vi "Main.vi"() -> ()   [LabVIEW 2012]
doc: "The top-level, or parent, VI for the Advanced Beam Line Electronics (ABLE) application. This VIs also acts as the main graphical user interface (GUI) for the application."
uses:
  ExperimentRun.ctl
  ExperimentRunTiming.ctl
  ExperimentRunDose.ctl
  ExperimentRunFluence.ctl
  ExperimentRunTotalCharge.ctl
  TemperatureAlarmSetup.ctl
  TemperatureAlarmStatus.ctl
  AboutButton.ctl
  UIActionQueueElement.ctl
  UIAction.ctl
  ExperimentActionQueueElement.ctl
  ExperimentAction.ctl
  Experiment.ctl
  Sample.ctl
  BeamLine.ctl
  BeamLineType.ctl
  BeamLineIon.ctl
  AlarmSetups.ctl
  AlarmSetup.ctl
  AlarmQueueElement.ctl
  AlarmAction.ctl
  <vilib>/Utility/error.llb/DialogType.ctl
  HardwareActionQueueElement.ctl
  HardwareAction.ctl
  libs/LV-Utilities/LV-Utilities.lvlib
panel:
  in  "SHOW ABOUT":T1
  in  "ALARMS":bool
  out "Runs":T2[](array[typedef])
  in  "EXPERIMENT":bool
  in  "OVERVIEW":bool
  in  "Tab Control":enum32{"Overview", "Experiment", "Alarms"}(tab)
  out "Overview Temperatures":dbl[][](graph)
  out "Overview Currents":dbl[][](graph)
  out "Beam Profile":cluster{"Waveform":dbl[], "Waveform":dbl[]}[](graph)
  out "DPA Rate":dbl format="%.3e"
  out "Flux":dbl format="%.3e"
  out "Average Flux":dbl format="%.3e"
  out "Average DPA Rate":dbl format="%.3e"
  out "Completed":dbl format="%.1f"
  out "Fluence":dbl format="%.3e"
  out "Dose":dbl format="%.3e"
  out "Total Charge":dbl format="%.3p"
  out "West Aperture":dbl format="%.1p"
  out "Beam Current":dbl format="%.1p"
  out "East Aperture":dbl format="%.1p"
  out "South Aperture":dbl format="%.1p"
  out "North Aperture":dbl format="%.1p"
  out "Overview Voltages":dbl(graph)
  out "Total Ion Energy":dbl format="%.3f"
  out "Terminal Voltage":dbl format="%.3p"
  out "Average":dbl format="%.1f"
  out "Temperature 3":dbl format="%.1f"
  out "Temperature 2":dbl format="%.1f"
  out "Temperature 1":dbl format="%.1f"
  out "Experiment Total Runs":u32
  in  "SHOW RUNS":bool
  out "Experiment Completed":dbl=nan format="%.1f"
  in  "Experiment Target Dose (dpa)":dbl=nan format="%.3e"
  in  "Experiment Project":string
  in  "Experiment Operator":string="Operator"
  in  "SELECT SRIM":bool
  in  "Experiment Sample SRIM Damage Peak (disp * ion / cm)":dbl=nan format="%.2e"
  in  "Experiment Beam Line Total Source Ion Energy (kV)":dbl=nan format="%.1f"
  in  "Experiment Beam Line Charge State":u8=1
  in  "Experiment Beam Line Ion":T7(ring)
  in  "Experiment Beam Line Type":T8(ring)
  in  "Experiment Sample Irradiation Area (cm^2)":dbl=nan format="%.4f"
  in  "Experiment Sample Density (g/cm^3)":dbl=nan format="%.3f"
  in  "Experiment Sample Molar Mass (g/mol)":dbl=nan format="%.3f"
  in  "Experiment Sample Name":string="Sample Name"
  in  "Experiment Sample Description":string="Sample Description"
  out "Experiment File Path":path
  out "Running?":bool
  in  "START EXPERIMENT":bool
  in  "CLOSE EXPERIMENT":bool
  in  "SAVE EXPERIMENT":bool
  in  "OPEN EXPERIMENT":bool
  in  "NEW EXPERIMENT":bool
  out "Temperature 2 Alarm Status":T9={"Actual (C)"=nan, "Activated?"=FALSE} {"Actual (C)" format="%.1f"}
  in  "Temperature 2 Alarm Setup":T10={"ENABLED"=FALSE, "High Limit (C)"=nan, "Low Limit (C)"=nan} {"Low Limit (C)" format="%.1f"; "High Limit (C)" format="%.1f"}
  out "Temperature 1 Alarm Status":T9={"Actual (C)"=nan, "Activated?"=FALSE} {"Actual (C)" format="%.1f"}
  in  "Temperature 1 Alarm Setup":T10={"ENABLED"=FALSE, "High Limit (C)"=nan, "Low Limit (C)"=nan} {"Low Limit (C)" format="%.1f"; "High Limit (C)" format="%.1f"}
  in  "Average Temperature Alarm Setup":T10={"ENABLED"=FALSE, "High Limit (C)"=nan, "Low Limit (C)"=nan} {"Low Limit (C)" format="%.1f"; "High Limit (C)" format="%.1f"}
  out "Average Temperature Alarm Status":T9={"Actual (C)"=nan, "Activated?"=FALSE} {"Actual (C)" format="%.1f"}
  in  "Temperature 3 Alarm Setup":T10={"ENABLED"=FALSE, "High Limit (C)"=nan, "Low Limit (C)"=nan} {"Low Limit (C)" format="%.1f"; "High Limit (C)" format="%.1f"}
  out "Temperature 3 Alarm Status":T9={"Actual (C)"=nan, "Activated?"=FALSE} {"Actual (C)" format="%.1f"}
  in  "DONE":bool
  # "Experiment"
  # "Currents"
  # "Voltages"
  # "Temperatures"
  # "RUNS"
  # "Total Runs"
  # "Completed (%)"
  # "Experiment"
  # "Target Dose"
  # "Project Description"
  # "Operator"
  # "SRIM"
  # "Damage Peak (D1)"
  # "Beam Line"
  # "Total Source Ion Energy"
  # "Ion"
  # "+"
  # "Type"
  # "Sample"
  # "Irradiation Area"
  # "Density"
  # "Molar Mass"
  # "Name"
  # "Description"
  # "Temperature 2"
  # "Actual"
  # "Low Limit"
  # "High Limit"
  # "Temperature 1"
  # "Actual"
  # "Low Limit"
  # "High Limit"
  # "Average Temperature"
  # "Low Limit"
  # "High Limit"
  # "Actual"
  # "Temperature 3"
  # "Low Limit"
  # "High Limit"
  # "Actual"
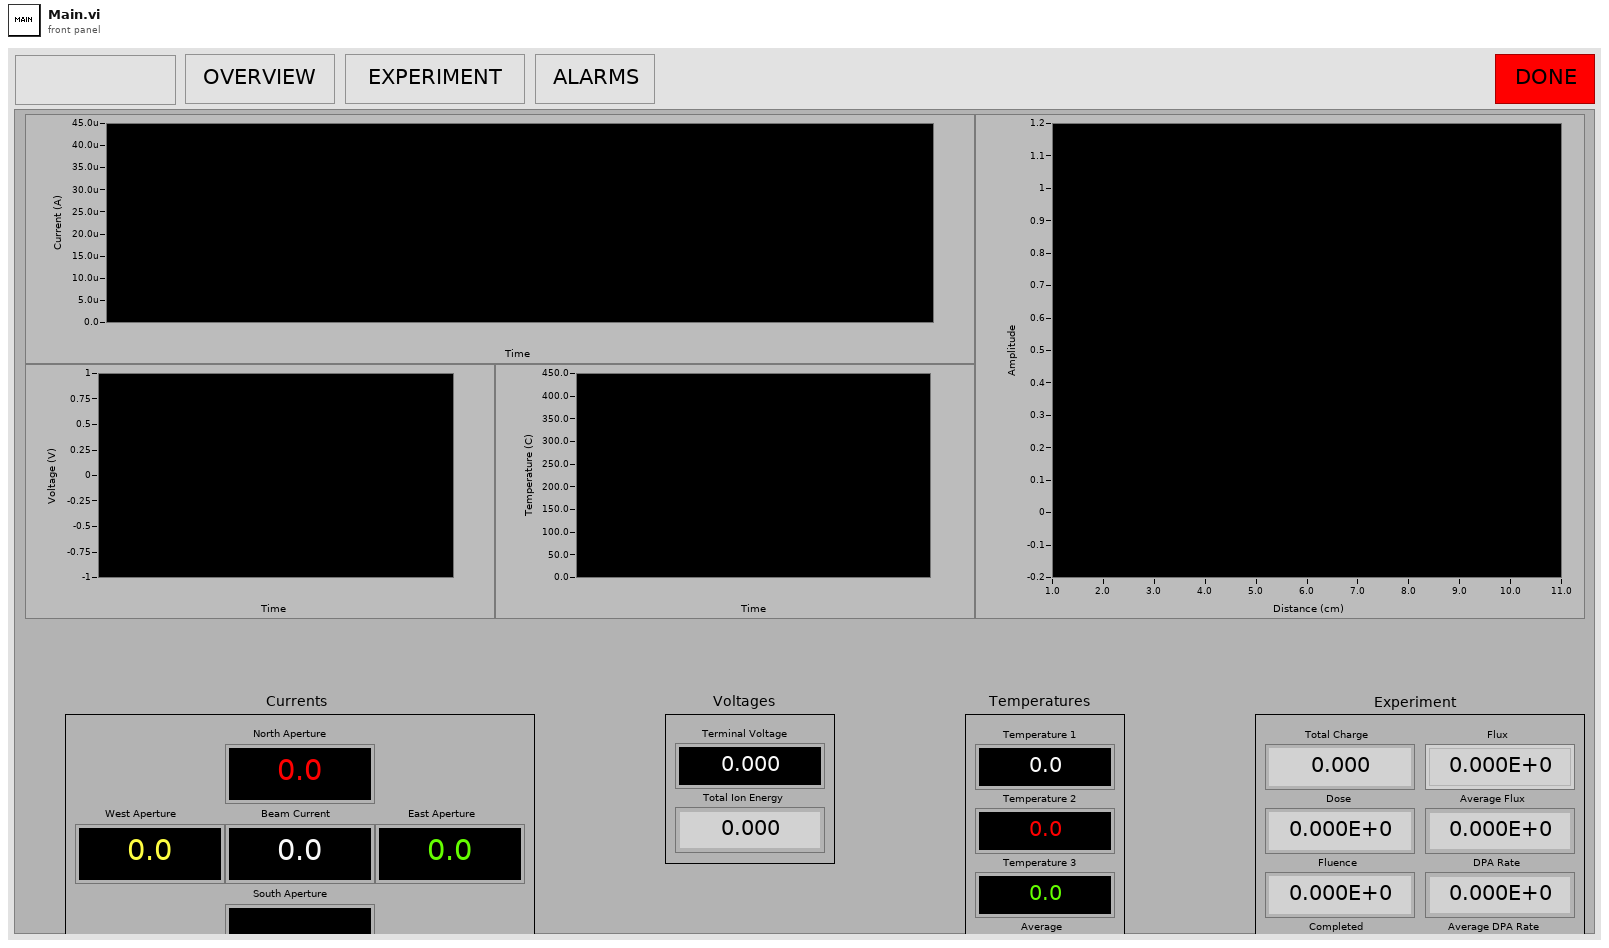
[diagram p1: front panel]
types:
  T1 = typedef "AboutButton.ctl" = bool
  T2 = typedef "ExperimentRun.ctl" = cluster{"Timing":T3, "Dose (dpa)":T4, "Fluence (ions/cm^2)":T5, "Total Charge (C)":T6}
  T3 = typedef "ExperimentRunTiming.ctl" = cluster{"Start":timestamp, "Stop":timestamp}
  T4 = typedef "ExperimentRunDose.ctl" = cluster{"Start":dbl, "Stop":dbl}
  T5 = typedef "ExperimentRunFluence.ctl" = cluster{"Start":dbl, "Stop":dbl}
  T6 = typedef "ExperimentRunTotalCharge.ctl" = cluster{"Start":dbl, "Stop":dbl}
  T7 = enum16{"H", "He", "C", "Fe", "Ni", "Pt", "Si", "Ag", "Au"}
  T8 = enum16{"Ion Beam Analysis", "Auxiliary", "Radiation Damage"}
  T9 = typedef "TemperatureAlarmStatus.ctl" = cluster{"Actual (C)":dbl, "Activated?":bool}
  T10 = typedef "TemperatureAlarmSetup.ctl" = cluster{"ENABLED":bool, "High Limit (C)":dbl, "Low Limit (C)":dbl}
  T11 = typedef "ABLEConfiguration.ctl" = cluster{"Display":T12, "Simulate Data?":bool, "Folder":T13, "Alarms":T14, "Keithley 6485":T15, "Keithley 6482":T16}
  T12 = typedef "DisplayConfiguration.ctl" = cluster{"Defualt Monitor":u16, "Center on Monitor?":bool, "Hardware Display Period (msec)":u32, "Experiment Display Period (msec)":u32}
  T13 = typedef "FolderConfiguration.ctl" = cluster{"Hardware Log":path, "Experiment Log":path, "Experiment":path, "SRIM Simulation":path}
  T14 = typedef "AlarmsConfiguration.ctl" = cluster{"Temperature Alarm Sound File":path, "Temperature Alarm Sound Delay (sec)":dbl}
  T15 = typedef "Keithley6485Configuration.ctl" = cluster{"GPIB IDs":u8[], "GPIB Board IDs":u8[], "Display On?":bool[], "Integration Rates":dbl[], "Auto Range?":bool[], "Ranges (A)":dbl[]}
  T16 = typedef "Keithley6482Configuration.ctl" = cluster{"GPIB IDs":u8[], "GPIB Board IDs":u8[], "Display On?":bool[], "Integration Rates":dbl[], "Auto Range?":bool[], "Ranges (A)":dbl[]}
  T17 = typedef "ABLEDataStructures.ctl" = cluster{"Hardware Display":refnum<notifier>, "BPM":refnum<notifier>, "Experiment Hardware":refnum<notifier>, "Experiment Display":refnum<notifier>, "Alarm Display":refnum<notifier>}
  T18 = typedef "ActionQueues.ctl" = cluster{"UI Action":refnum<queue>, "Hardware Action":refnum<queue>, "Experiment Action":refnum<queue>, "Alarm Action":refnum<queue>}
  T19 = typedef "HardwareDisplayData.ctl" = cluster{"Temperatures (C)":dbl[], "Terminal Voltage (MeV)":dbl, "Currents (A)":dbl[]}
  T20 = typedef "AlarmData.ctl" = cluster{"Temperature":T21[]}
  T21 = typedef "AlarmDatum.ctl" = cluster{"Actual":dbl, "Activated?":bool}
  T22 = typedef "ExperimentData.ctl" = cluster{"Flux (ions/s * cm^2)":dbl, "Average Flux (ions/s * cm^2)":dbl, "DPA Rate":dbl, "Average DPA Rate":dbl, "Total Ion Energy (MeV)":dbl, "Total Charge (C)":dbl, "Dose (DPA)":dbl, "Fluence (ions/cm^2)":dbl, "Percent Complete (%)":dbl, "Duration (sec)":dbl}
  T23 = typedef "UIActionQueueElement.ctl" = cluster{"Action":T24, "Data":variant}
  T24 = typedef "UIAction.ctl" = enum16{"Initalize", "Create Experiment", "Created", "Read Experiment Controls", "Read Alarm Controls", "Loaded", "Save Experiment", "Saved", "Write Experiment Controls", "Read Experiment", "Read", "Start Experiment", "Started", "Stop Experiment", "Stopped", "Close Experiment", "Closed", "SRIM", "Error", "Shutdown"}
  T25 = enum8{"Enabled", "Disabled", "Disabled and Grayed Out"}
  T26 = typedef "ExperimentActionQueueElement.ctl" = cluster{"Action":T27, "Data":variant}
  T27 = typedef "ExperimentAction.ctl" = enum16{"Initialize", "Create", "Read", "Load", "Start", "Run", "Stop", "Save", "Shutdown"}
  T28 = typedef "BeamLine.ctl" = cluster{"Type":T29, "Ion":T30, "Charge State":u8, "Total Source Ion Energy (kV)":dbl}
  T29 = typedef "BeamLineType.ctl" = enum16{"Ion Beam Analysis", "Auxiliary", "Radiation Damage"}
  T30 = typedef "BeamLineIon.ctl" = enum16{"H", "He", "C", "Fe", "Ni", "Pt", "Si", "Ag", "Au"}
  T31 = typedef "Sample.ctl" = cluster{"Name":string, "Description":string, "Molar Mass (g/mol)":dbl, "Density (g/cm^3)":dbl, "Irradiation Area (cm^2)":dbl, "SRIM Damage Peak (disp * ions/cm)":dbl}
  T32 = typedef "Experiment.ctl" = cluster{"File Path":path, "Operator":string, "Project":string, "Target Dose (dpa)":dbl, "Sample":T31, "Beam Line":T28, "Runs":T2[]}
  T33 = typedef "AlarmQueueElement.ctl" = cluster{"Action":T34, "Data":variant}
  T34 = typedef "AlarmAction.ctl" = enum16{"Initialize", "Load", "Check", "Shutdown"}
  T35 = typedef "AlarmSetups.ctl" = cluster{"Temperature":T36[]}
  T36 = typedef "AlarmSetup.ctl" = cluster{"ENABLED":bool, "High Limit":dbl, "Low Limit":dbl}
  T37 = typedef "HardwareActionQueueElement.ctl" = cluster{"Action":T38, "Data":variant}
  T38 = typedef "HardwareAction.ctl" = enum16{"Initialize", "Collect", "Shutdown"}
  T39 = typedef "DialogType.ctl" = u16
  T40 = typedef "BPM.ctl" = cluster{dbl[], "Beam Profile":dbl[]}[]
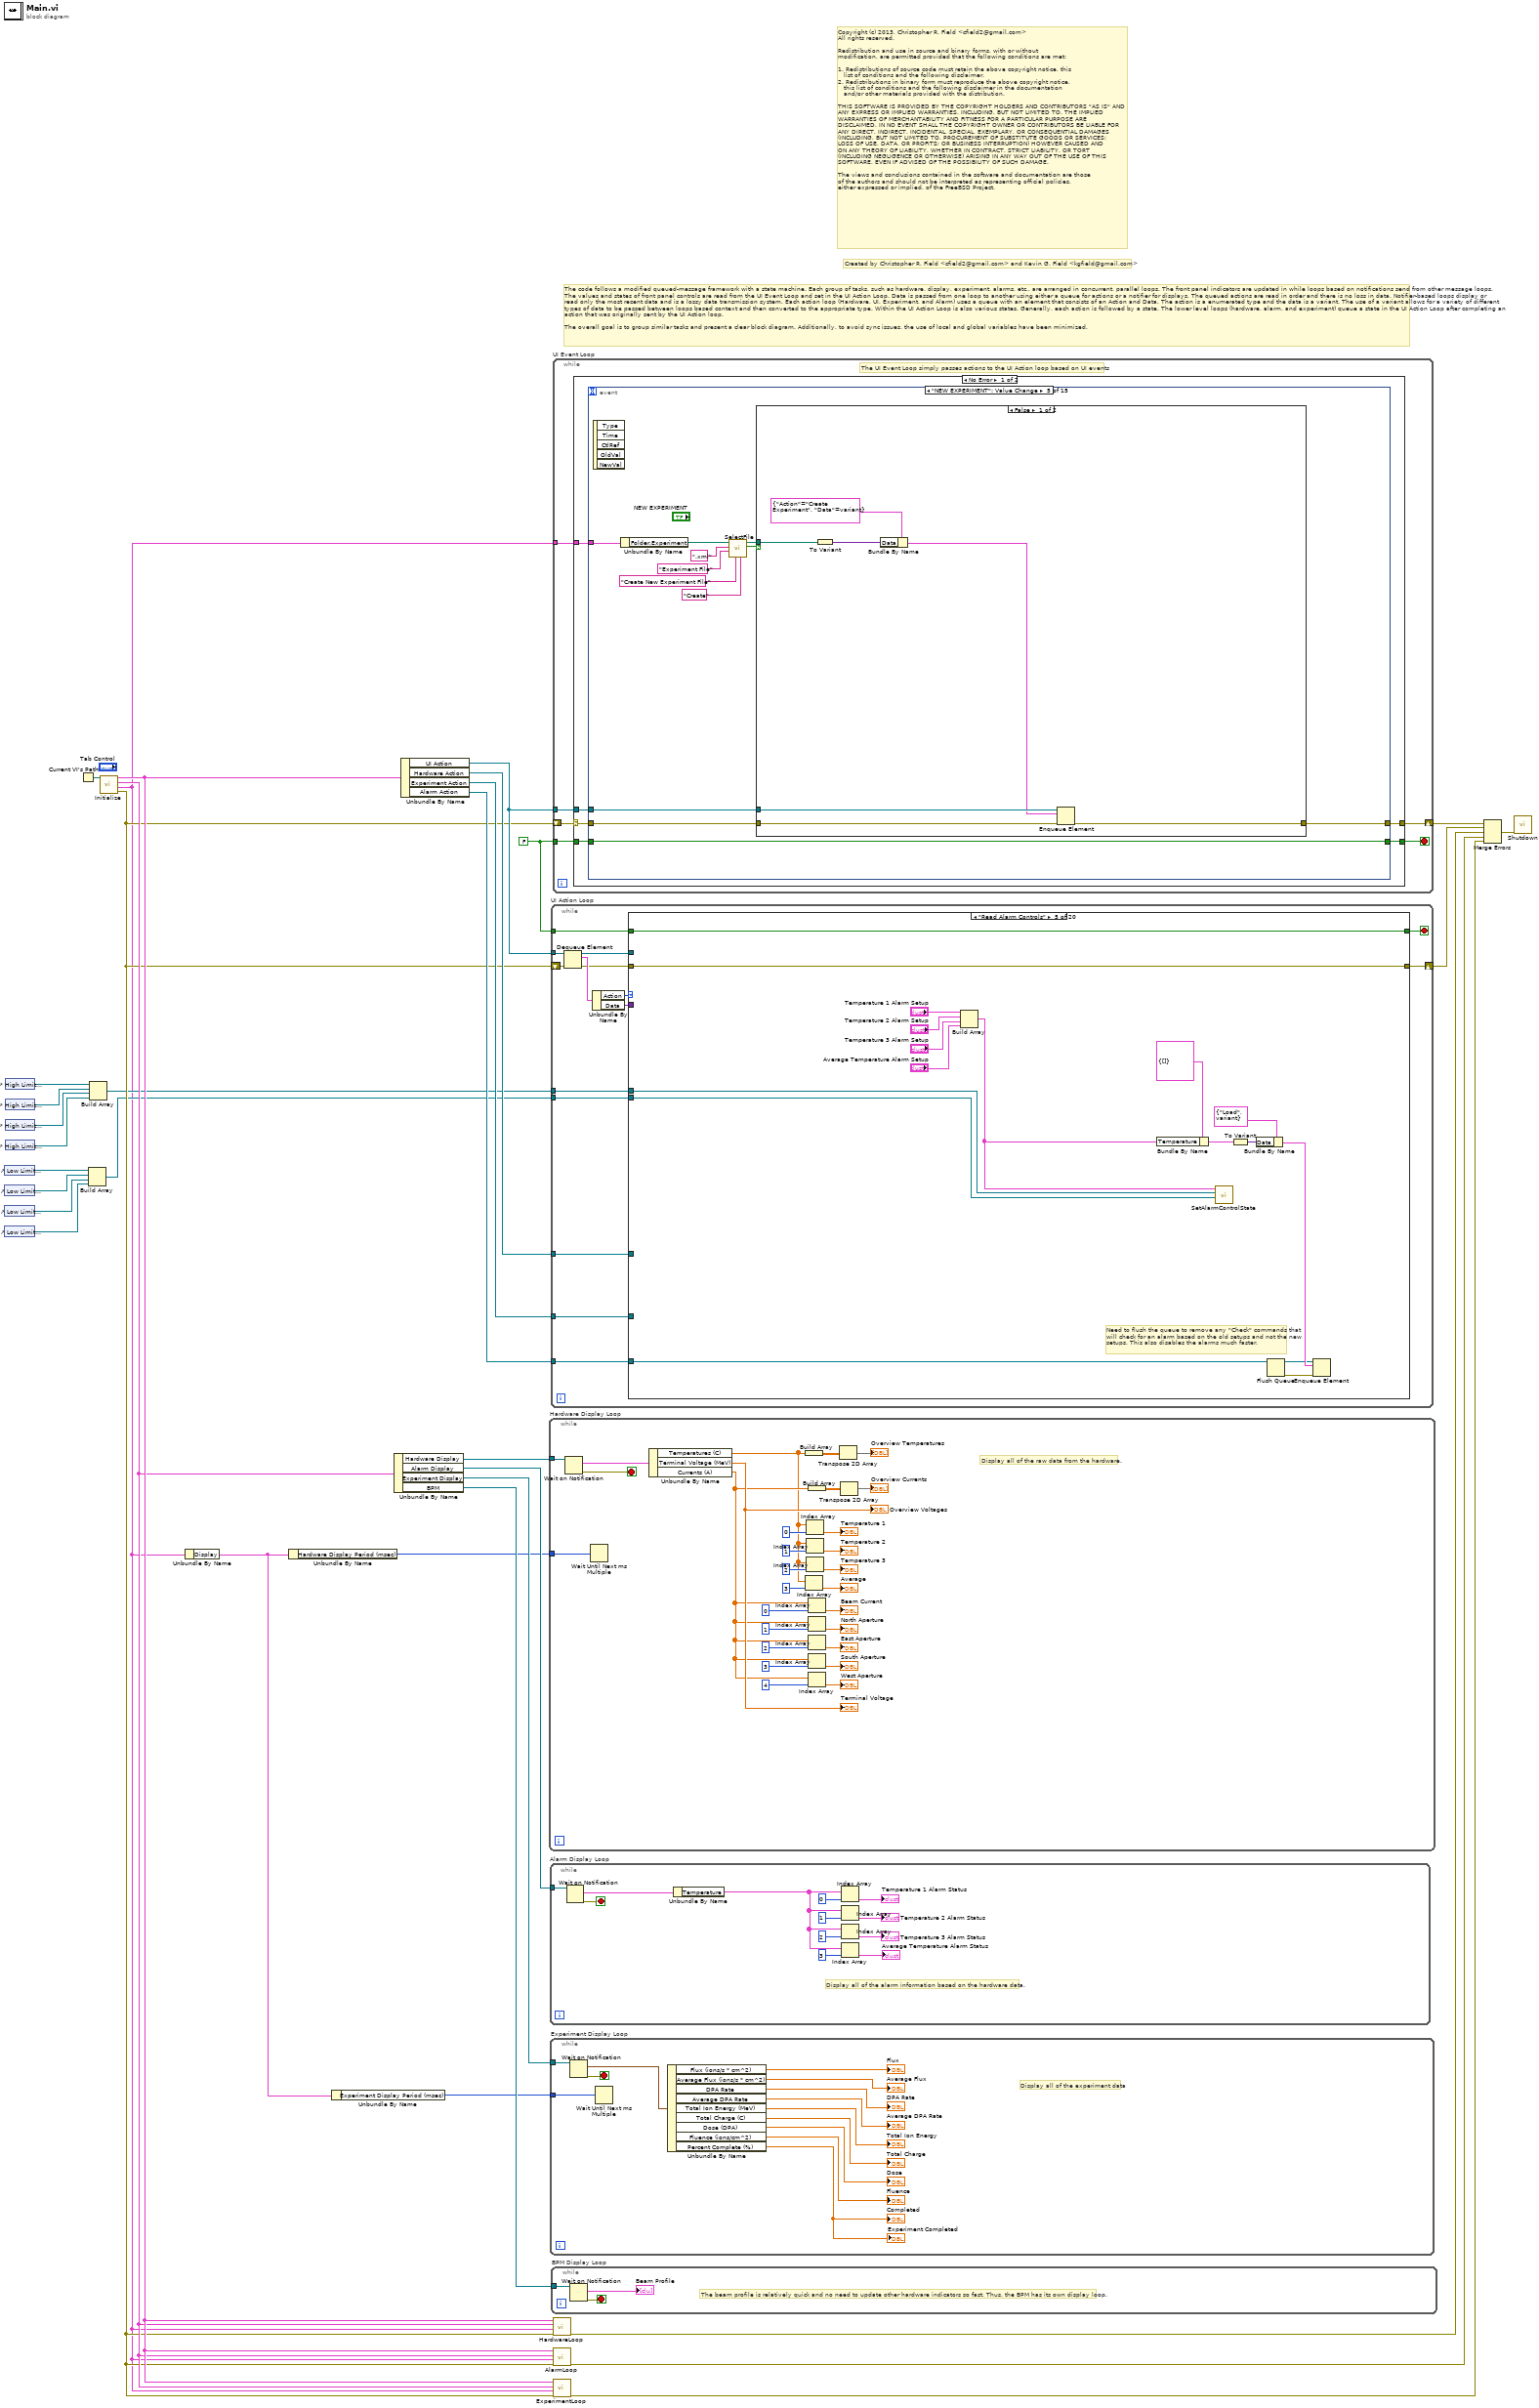
[diagram p0: block diagram]
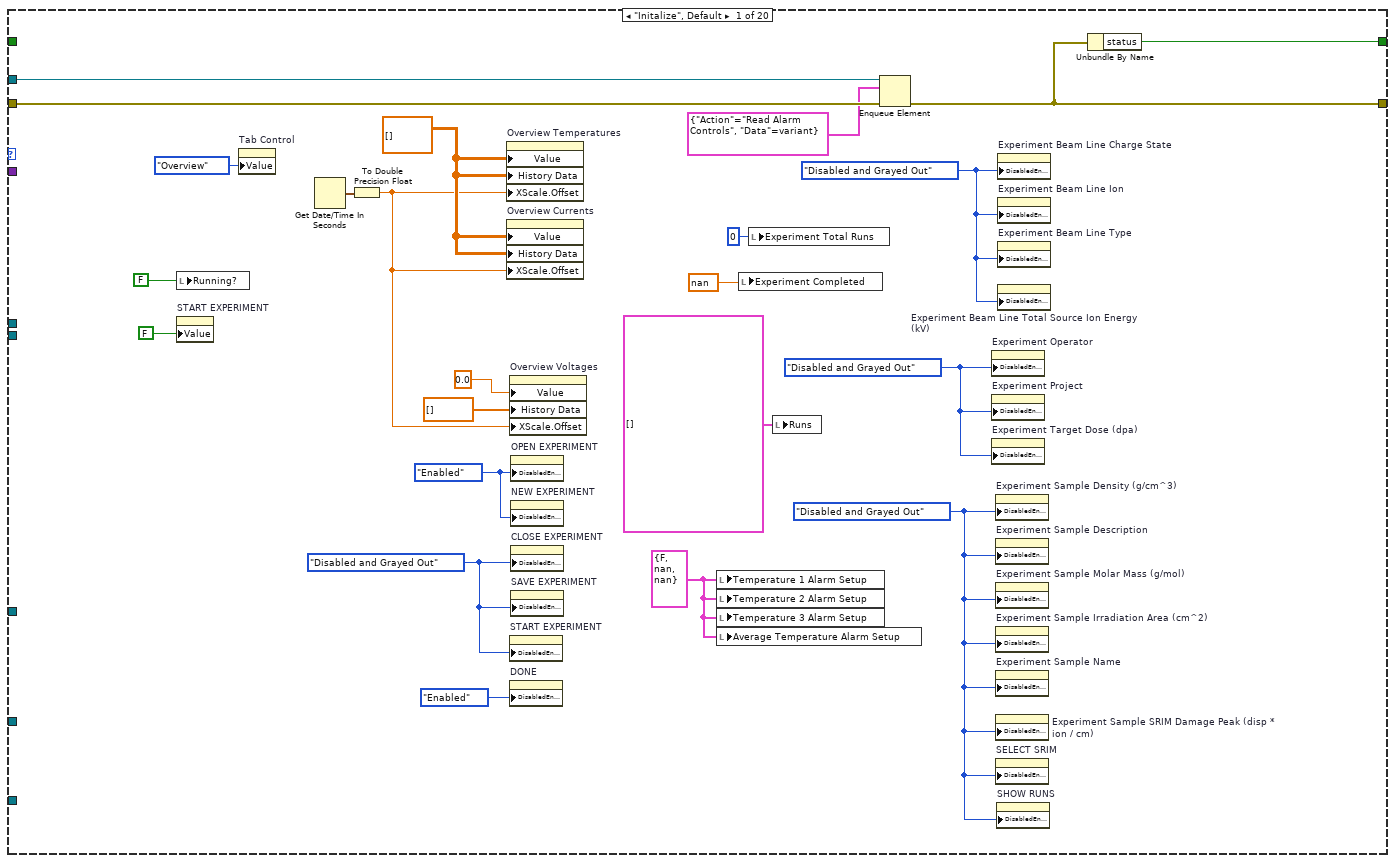
[diagram p2: hidden frame]
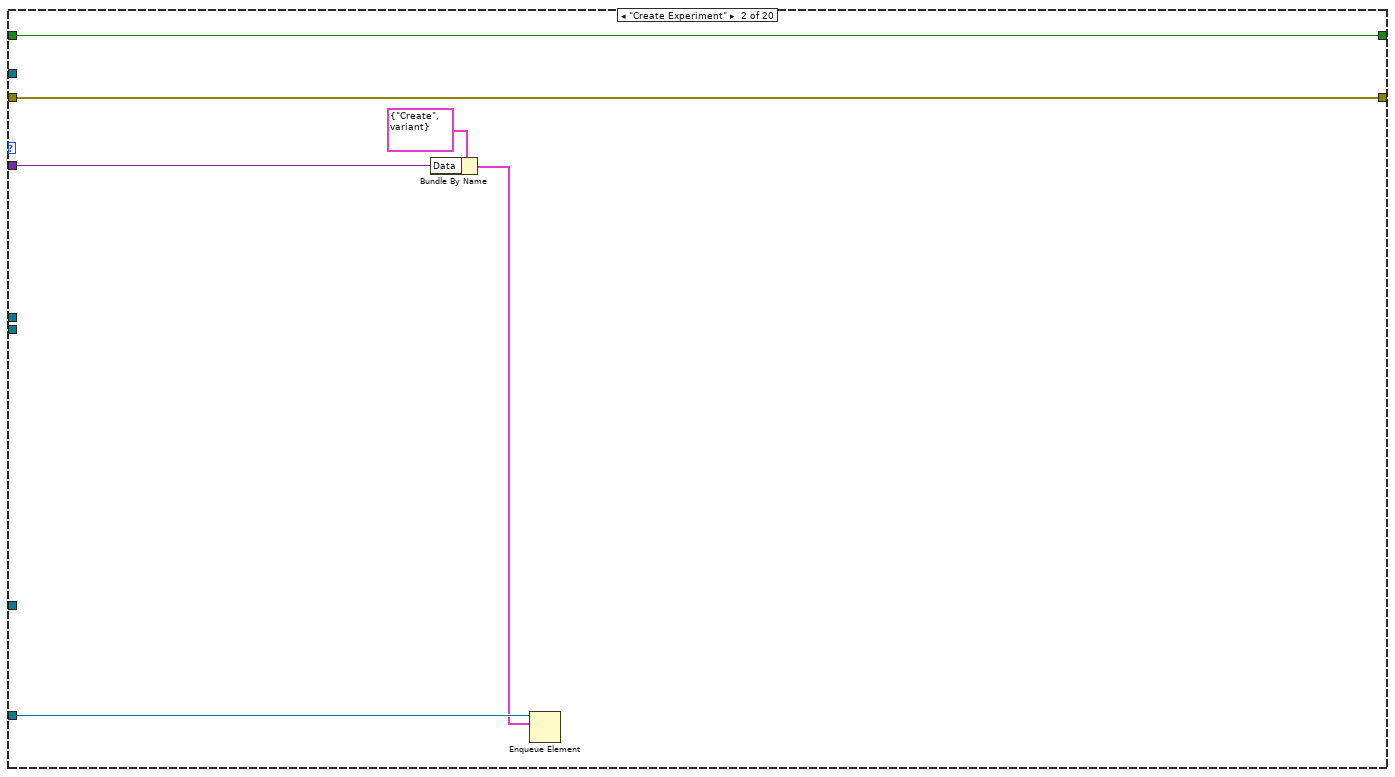
[diagram p3: hidden frame]
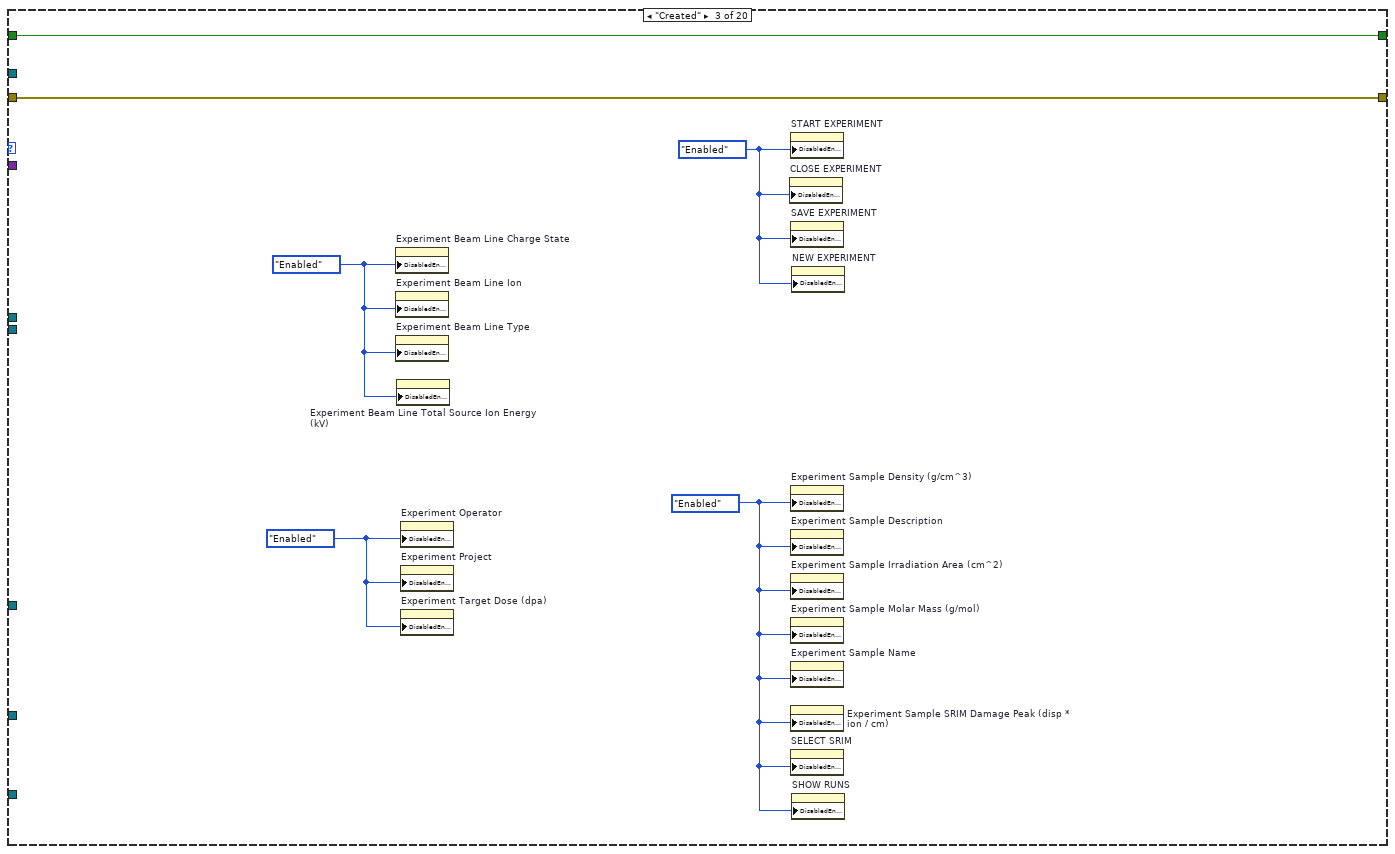
[diagram p4: hidden frame]
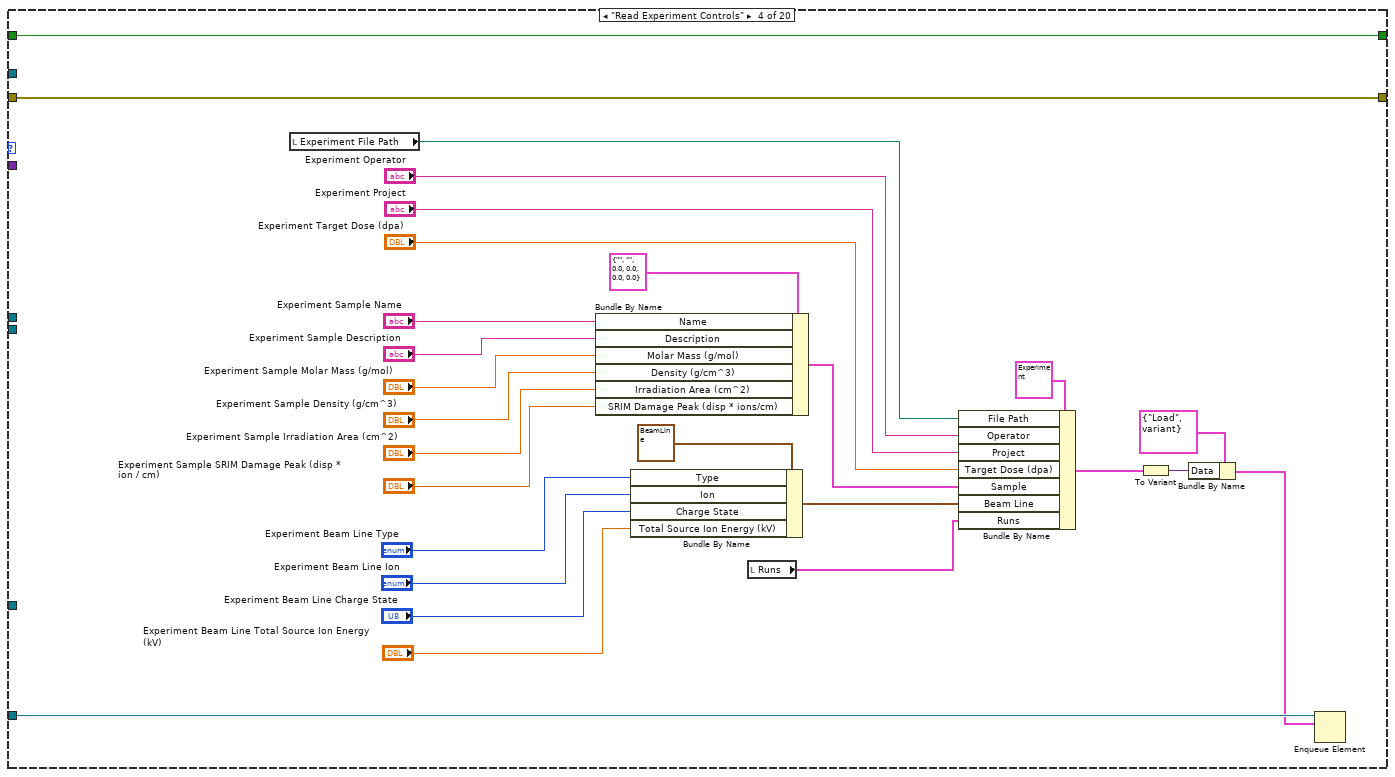
[diagram p5: hidden frame]
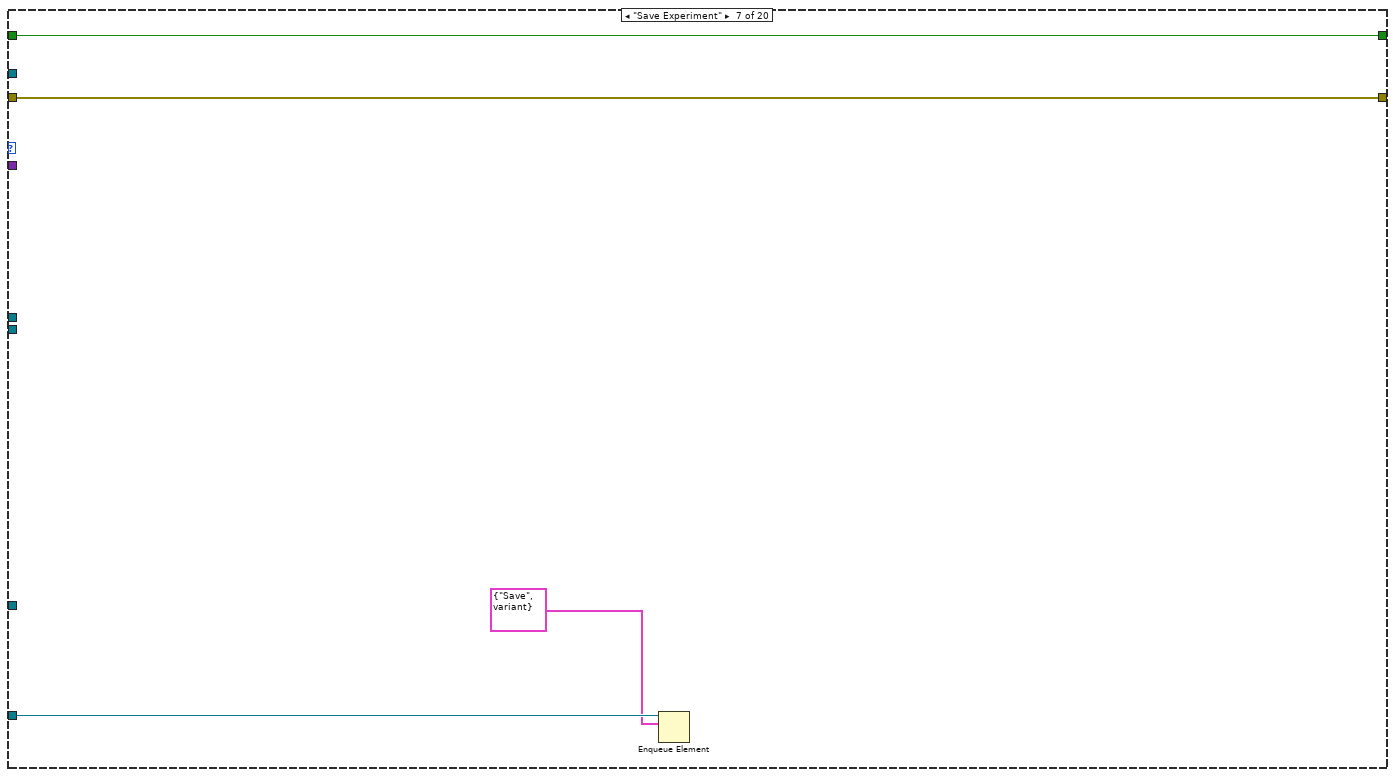
[diagram p7: hidden frame]
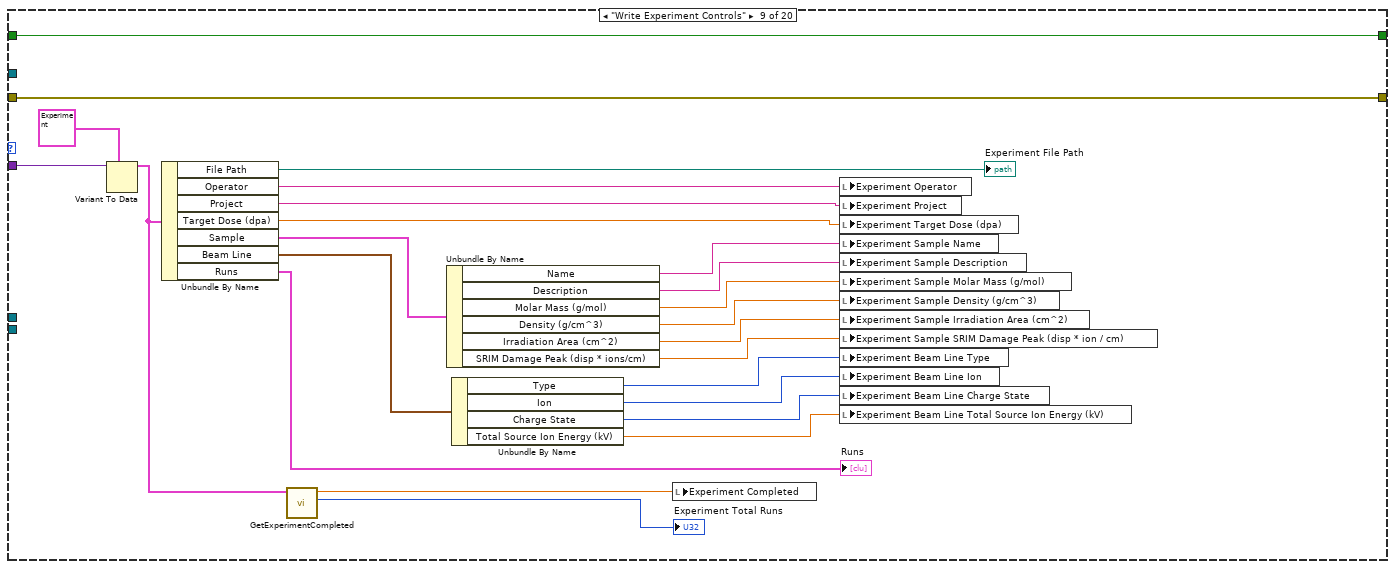
[diagram p9: hidden frame]
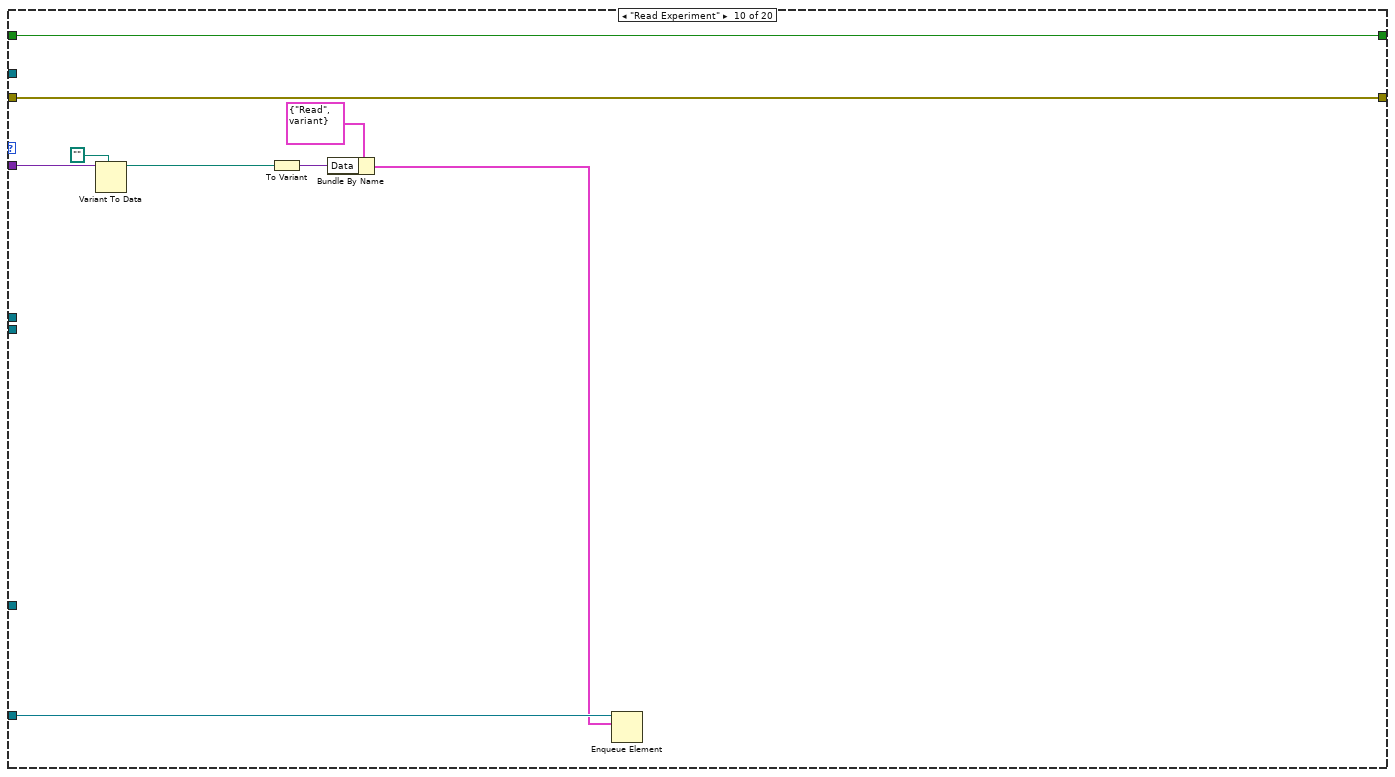
[diagram p10: hidden frame]
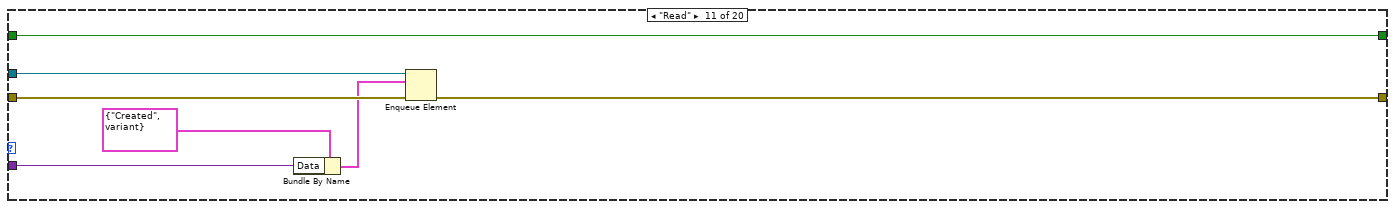
[diagram p11: hidden frame]
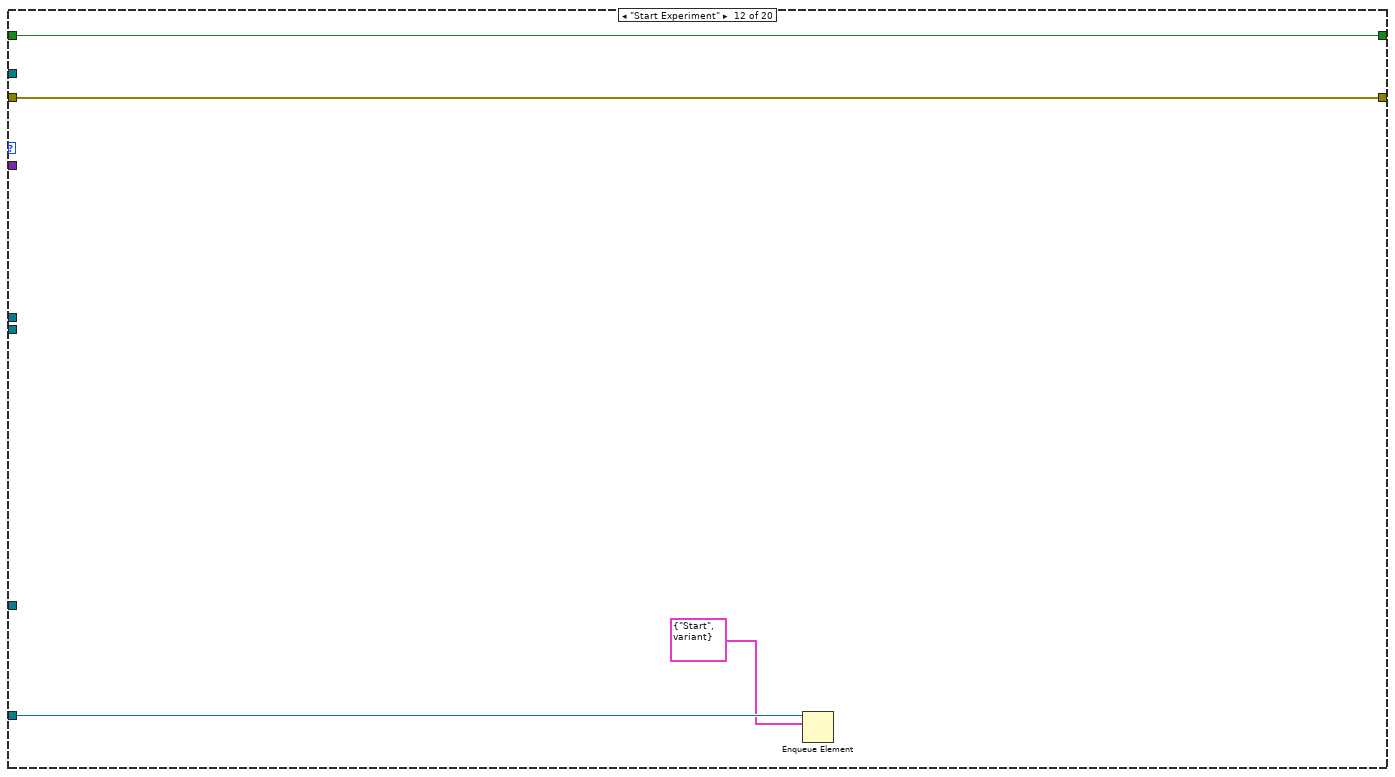
[diagram p12: hidden frame]
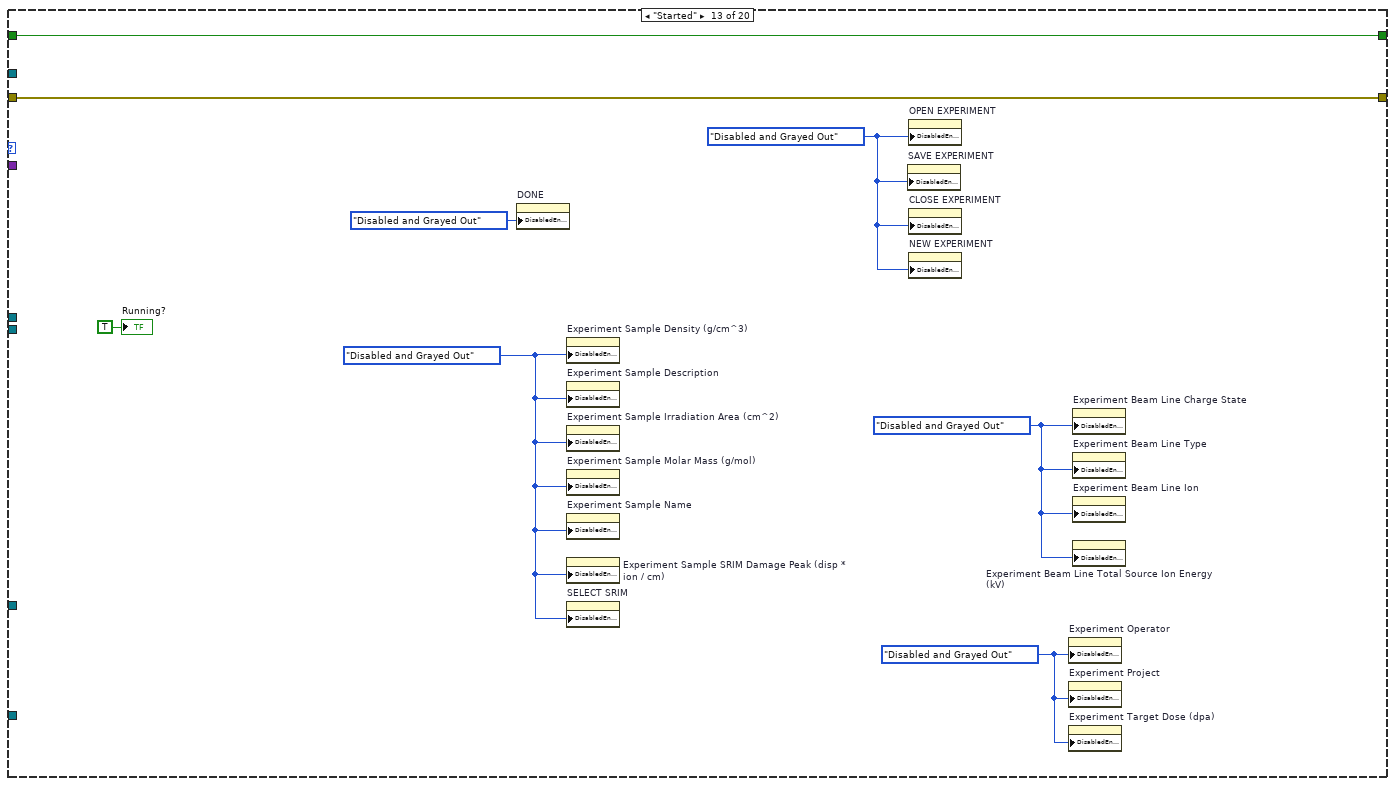
[diagram p13: hidden frame]
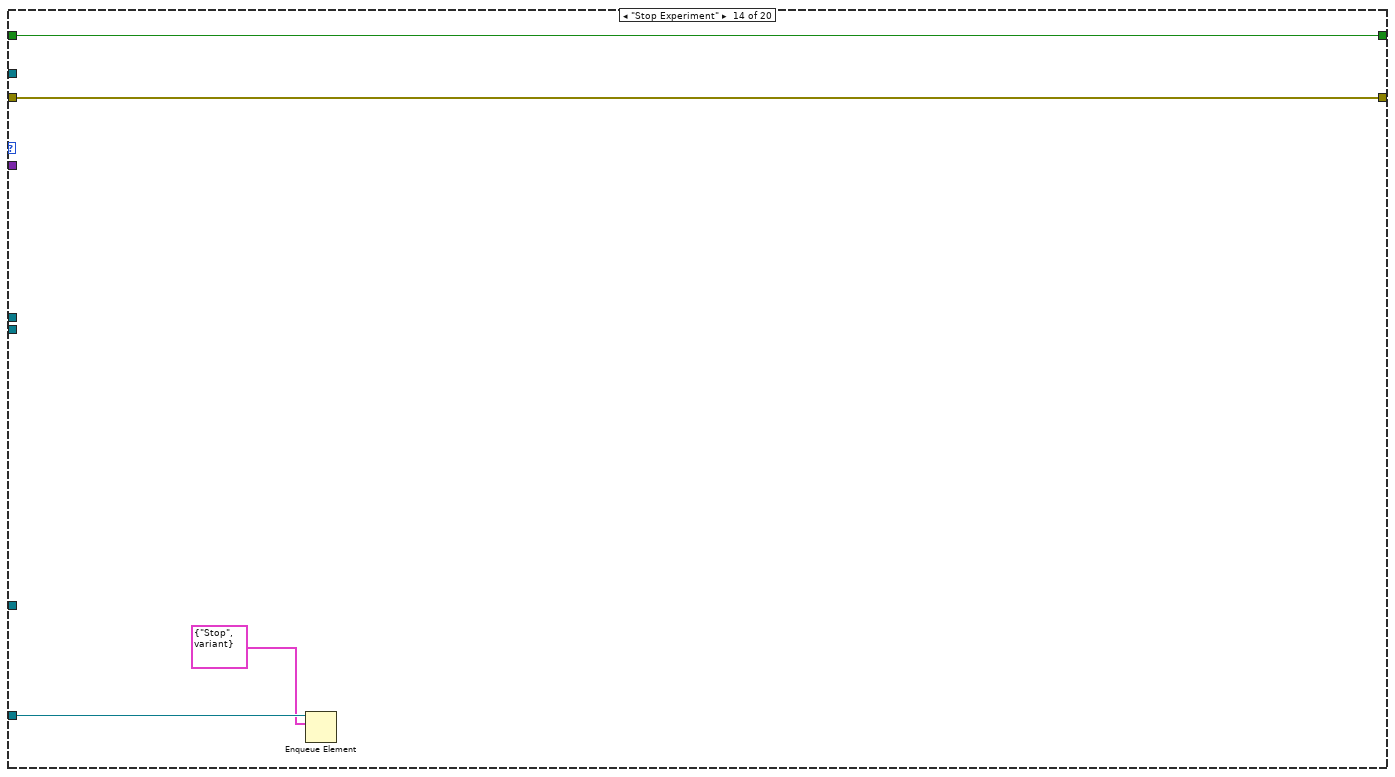
[diagram p14: hidden frame]
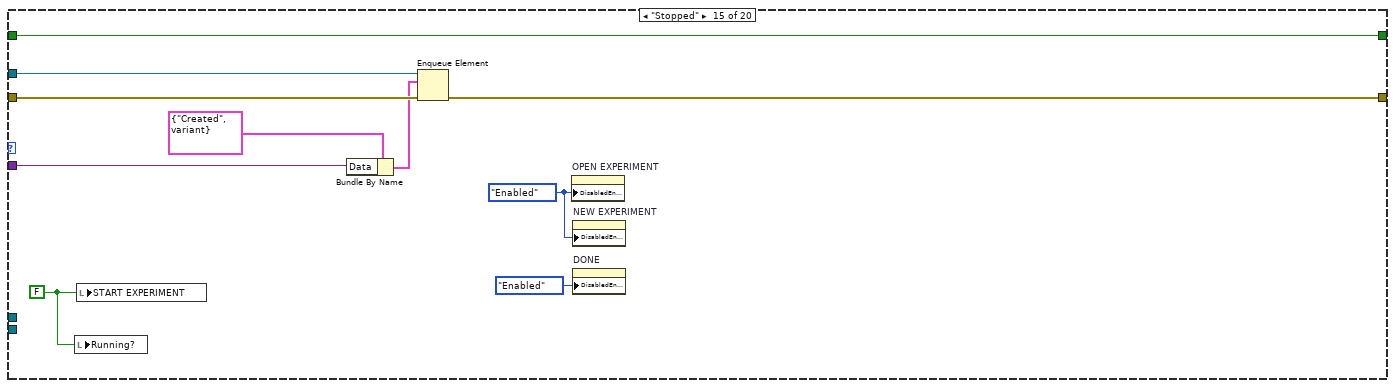
[diagram p15: hidden frame]
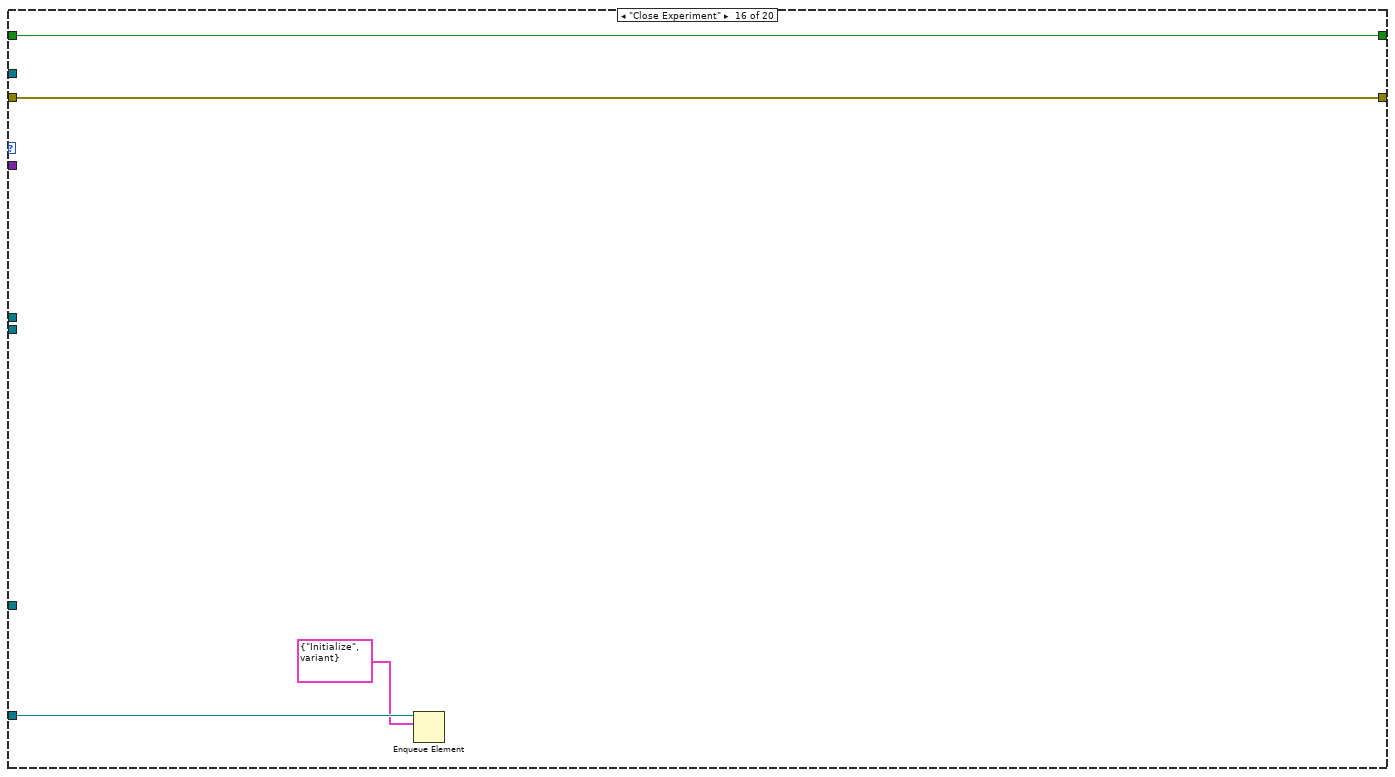
[diagram p16: hidden frame]
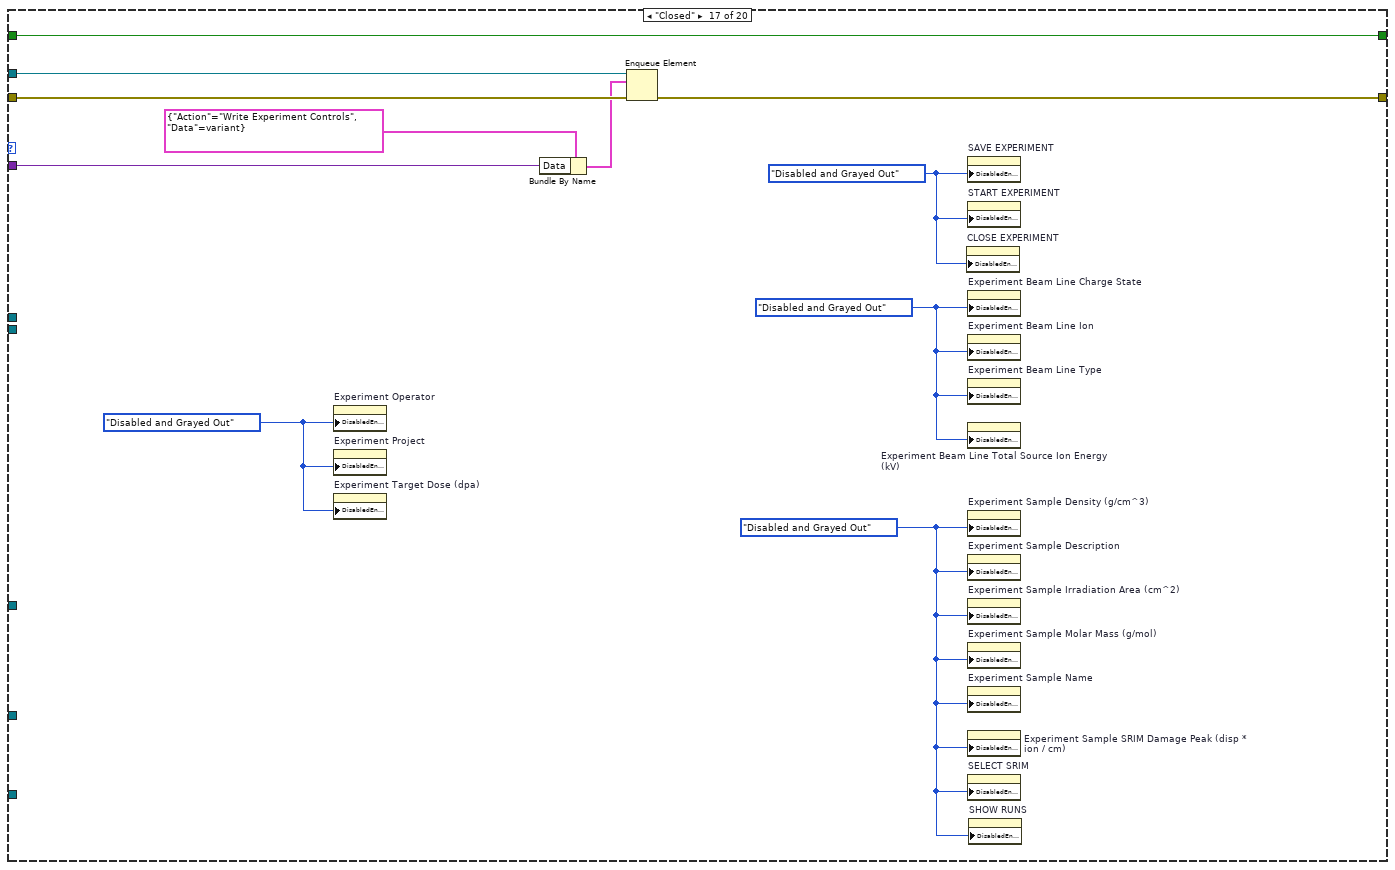
[diagram p17: hidden frame]
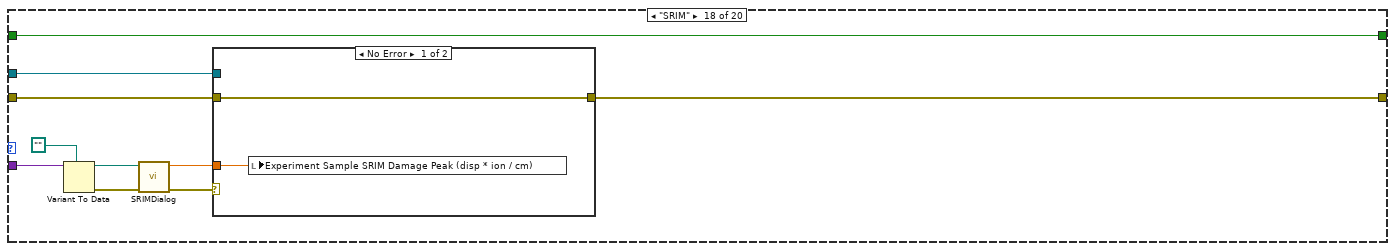
[diagram p18: hidden frame]
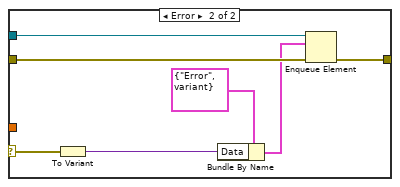
[diagram p19: hidden frame]
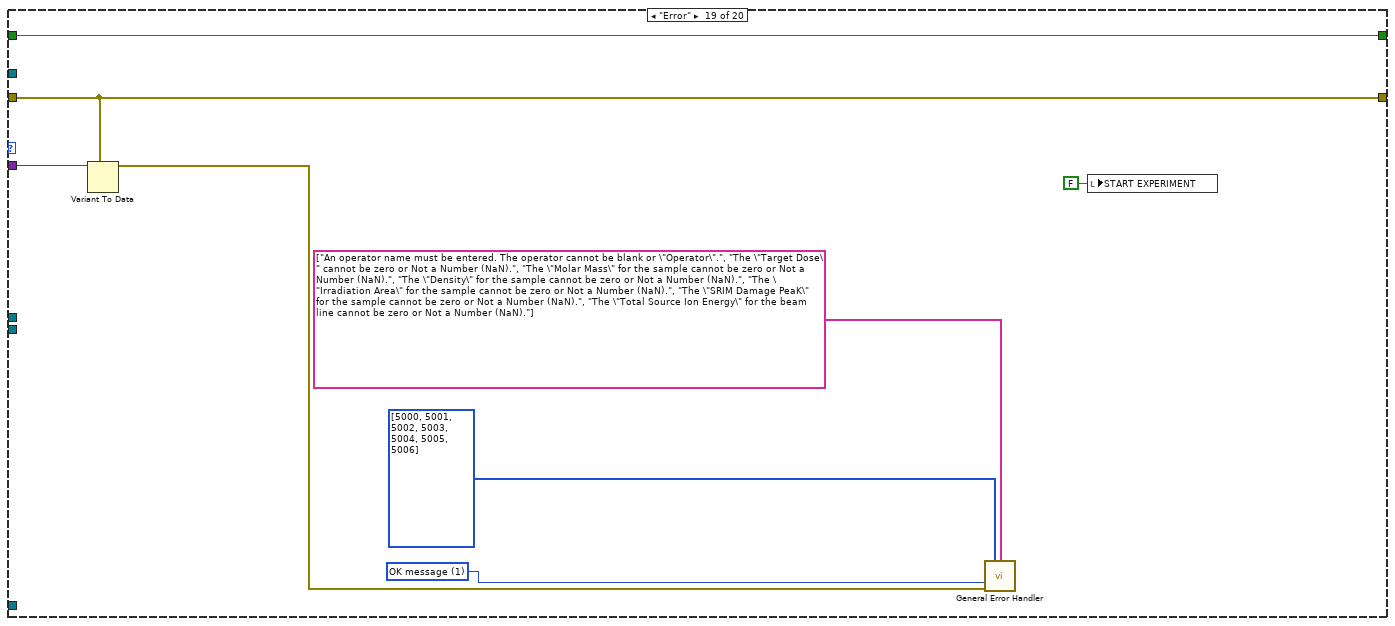
[diagram p20: hidden frame]
diagram:
  w33 = FALSE
  # "Copyright (c) 2013, Christopher R. Field <cfield2@gmail.com>\nAll rights reserved.\n\nRedistribution and use in source and binary forms, with or without\nmodification, are permitted provided that the following conditions are met: \n\n1. Redistributions of source code must retain the above copyright notice, this\n   list of conditions and the following disclaimer. \n2. Redistributions in binary form must reproduce the above copyright notice,\n   this list of conditions and the following disclaimer in the documentation\n   and/or other materials provided with the distribution. \n\nTHIS SOFTWARE IS PROVIDED BY THE COPYRIGHT HOLDERS AND CONTRIBUTORS \"AS IS\" AND\nANY EXPRESS OR IMPLIED WARRANTIES, INCLUDING, BUT NOT LIMITED TO, THE IMPLIED\nWARRANTIES OF MERCHANTABILITY AND FITNESS FOR A PARTICULAR PURPOSE ARE\nDISCLAIMED. IN NO EVENT SHALL THE COPYRIGHT OWNER OR CONTRIBUTORS BE LIABLE FOR\nANY DIRECT, INDIRECT, INCIDENTAL, SPECIAL, EXEMPLARY, OR CONSEQUENTIAL DAMAGES\n(INCLUDING, BUT NOT LIMITED TO, PROCUREMENT OF SUBSTITUTE GOODS OR SERVICES;\nLOSS OF USE, DATA, OR PROFITS; OR BUSINESS INTERRUPTION) HOWEVER CAUSED AND\nON ANY THEORY OF LIABILITY, WHETHER IN CONTRACT, STRICT LIABILITY, OR TORT\n(INCLUDING NEGLIGENCE OR OTHERWISE) ARISING IN ANY WAY OUT OF THE USE OF THIS\nSOFTWARE, EVEN IF ADVISED OF THE POSSIBILITY OF SUCH DAMAGE.\n\nThe views and conclusions contained in the software and documentation are those\nof the authors and should not be interpreted as representing official policies, \neither expressed or implied, of the FreeBSD Project."
  # "Created by Christopher R. Field <cfield2@gmail.com> and Kevin G. Field <kgfield@gmail.com>"
  # "The code follows a modified queued-message framework with a state machine. Each group of tasks, such as hardware, display, experiment, alarms, etc., are arranged in concurrent, parallel loops. The front panel indicators are updated in while loops based on notifications send from other message loops. The values and states of front panel controls are read from the UI Event Loop and set in the UI Action Loop. Data is passed from one loop to another using either a queue for actions or a notifier for displays. The queued actions are read in order and there is no loss in data. Notifier-based loops display or read only the most recent data and is a lossy data transmission system. Each action loop (Hardware, UI, Experiment, and Alarm) uses a queue with an element that consists of an Action and Data. The action is a enumerated type and the data is a variant. The use of a variant allows for a variety of different types of data to be passed between loops based context and then converted to the appropriate type. Within the UI Action Loop is also various states. Generally, each action is followed by a state. The lower level loops (hardware, alarm, and experiment) queue a state in the UI Action Loop after completing an action that was originally sent by the UI Action loop.\n\nThe overall goal is to group similar tasks and present a clear block diagram. Additionally, to avoid sync issues, the use of local and global variables have been minimized."
  n1 = control-ref of="Low Limit (C)"() -> (w7:refnum<vi>)
  n2 = control-ref of="Low Limit (C)"() -> (w8:refnum<vi>)
  n3 = control-ref of="Low Limit (C)"() -> (w9:refnum<vi>)
  n4 = control-ref of="Low Limit (C)"() -> (w10:refnum<vi>)
  n5 = control-ref of="High Limit (C)"() -> (w11:refnum<vi>)
  n6 = control-ref of="High Limit (C)"() -> (w12:refnum<vi>)
  n7 = control-ref of="High Limit (C)"() -> (w13:refnum<vi>)
  n8 = control-ref of="High Limit (C)"() -> (w14:refnum<vi>)
  n9 = Current VI's Path() -> (path=w32:path)
  n10 = Build Array(w7, w8, w9, w10) -> (w5:refnum<vi>[])
  n11 = Build Array(w11, w12, w13, w14) -> (w6:refnum<vi>[])
  n12 = call "Initialize.vi"("VI Path"=w32) -> ("Error Out"=w17:errorcluster, "ABLE Configuration"=w4:T11, "ABLE Data Structures"=w18:T17, "Action Queues"=w19:T18)  [unwired: 7 in]
  n13 = Unbundle By Name(w4) -> ("Display"=w2:T12)
  n14 = Unbundle By Name(w2) -> ("Hardware Display Period (msec)"=w3:u32)
  n15 = Unbundle By Name(w2) -> ("Experiment Display Period (msec)"=w1:u32)
  n16 = Unbundle By Name(w18) -> ("Hardware Display"=w22:refnum<notifier>, "Alarm Display"=w21:refnum<notifier>, "Experiment Display"=w24:refnum<notifier>, "BPM"=w23:refnum<notifier>)
  n17 = Unbundle By Name(w19) -> ("UI Action"=w27:refnum<queue>, "Hardware Action"=w26:refnum<queue>, "Experiment Action"=w25:refnum<queue>, "Alarm Action"=w20:refnum<queue>)
  n18 = while "Hardware Display Loop" {
    tunnel: w22 -> [w41]
    tunnel: w3 -> [w34]
    stop <- w36 stop-if-true
    # "Display all of the raw data from the hardware."
    n19 = Wait on Notification(notifier=w41) -> (notification=w62:T19, error out=w36:errorcluster)  [unwired: 3 in, 2 out]
    n20 = Wait Until Next ms Multiple(millisecond multiple=w34) -> ()  [unwired: 1 out]
    n21 = Unbundle By Name(w62) -> ("Temperatures (C)"=w35:dbl[], "Terminal Voltage (MeV)"=→"Overview Voltages" →"Terminal Voltage":dbl, "Currents (A)"=w48:dbl[])
    n22 = Build Array(w35) -> (w50:dbl[][])
    n23 = Index Array(array=w35, index=3) -> (element=→"Average":dbl)
    n24 = Index Array(array=w35, index=0) -> (element=→"Temperature 1":dbl)
    n25 = Index Array(array=w35, index=1) -> (element=→"Temperature 2":dbl)
    n26 = Index Array(array=w35, index=2) -> (element=→"Temperature 3":dbl)
    n27 = Build Array(w48) -> (w47:dbl[][])
    n28 = Index Array(array=w48, index=3) -> (element=→"South Aperture":dbl)
    n29 = Index Array(array=w48, index=4) -> (element=→"West Aperture":dbl)
    n30 = Index Array(array=w48, index=0) -> (element=→"Beam Current":dbl)
    n31 = Index Array(array=w48, index=1) -> (element=→"North Aperture":dbl)
    n32 = Index Array(array=w48, index=2) -> (element=→"East Aperture":dbl)
    n33 = Transpose 2D Array(2D array=w50) -> (transposed array=→"Overview Temperatures":dbl[][])
    n34 = Transpose 2D Array(2D array=w47) -> (transposed array=→"Overview Currents":dbl[][])
  }
  n35 = while "Alarm Display Loop" {
    tunnel: w21 -> [w65]
    stop <- w74 stop-if-true
    # "Display all of the alarm information based on the hardware data."
    n36 = Wait on Notification(notifier=w65) -> (notification=w64:T20, error out=w74:errorcluster)  [unwired: 3 in, 2 out]
    n37 = Unbundle By Name(w64) -> ("Temperature"=w63:T21[])
    n38 = Index Array(array=w63, index=3) -> (element=→"Average Temperature Alarm Status":T21)
    n39 = Index Array(array=w63, index=0) -> (element=→"Temperature 1 Alarm Status":T21)
    n40 = Index Array(array=w63, index=1) -> (element=→"Temperature 2 Alarm Status":T21)
    n41 = Index Array(array=w63, index=2) -> (element=→"Temperature 3 Alarm Status":T21)
  }
  n42 = while "Experiment Display Loop" {
    tunnel: w24 -> [w86]
    tunnel: w1 -> [w75]
    stop <- w87 stop-if-true
    # "Display all of the experiment data"
    n43 = Wait on Notification(notifier=w86) -> (notification=w85:T22, error out=w87:errorcluster)  [unwired: 3 in, 2 out]
    n44 = Wait Until Next ms Multiple(millisecond multiple=w75) -> ()  [unwired: 1 out]
    n45 = Unbundle By Name(w85) -> ("Flux (ions/s * cm^2)"=→"Flux":dbl, "Average Flux (ions/s * cm^2)"=→"Average Flux":dbl, "DPA Rate"=→"DPA Rate":dbl, "Average DPA Rate"=→"Average DPA Rate":dbl, "Total Ion Energy (MeV)"=→"Total Ion Energy":dbl, "Total Charge (C)"=→"Total Charge":dbl, "Dose (DPA)"=→"Dose":dbl, "Fluence (ions/cm^2)"=→"Fluence":dbl, "Percent Complete (%)"=→"Completed" →"Experiment Completed":dbl)
  }
  n46 = while "UI Action Loop" {
    tunnel: w33 -> [w102]
    shift-right: [w94] -> w30
    shift-left: w17 -> [w98]
    tunnel: w27 -> [w93]
    tunnel: w26 -> [w92]
    tunnel: w25 -> [w91]
    tunnel: w20 -> [w90]
    tunnel: w6 -> [w89]
    tunnel: w5 -> [w88]
    stop <- w95 stop-if-true
    n47 = Dequeue Element(queue=w93, error in (no error)=w98) -> (queue out=w97:refnum<queue>, element=w101:T23, error out=w96:errorcluster)  [unwired: 1 in, 1 out]
    n48 = Unbundle By Name(w101) -> ("Action"=w100:T24, "Data"=w99:variant)
    n49 = case shown="\"Read Alarm Controls\"" w100 {
      tunnel: w102 -> [_ w131 w137 w164 w181 w183 w187 w189 w213 w222 w229 w233 w241 w245 w255 w259 w270 w280 w297 w320]
      tunnel: w99 -> [_ w126 _ _ _ _ _ _ w198 w221 w224 _ _ _ w248 _ w265 w279 w296 _]
      tunnel: w97 -> [w106 _ _ _ _ _ _ _ _ _ w228 _ _ _ w252 _ w269 w271 _ w311]
      tunnel: w96 -> [w105 w130 w133 w162 w180 w182 w186 w188 w212 w219 w227 w232 w235 w243 w250 w258 w268 w273 w295 w310]
      tunnel: [w107 w131 w137 w164 w181 w183 w187 w189 w213 w222 w229 w233 w241 w245 w255 w259 w270 w280 w297 w319] -> w95
      tunnel: [w104 w130 w133 w162 w180 w182 w186 w188 w212 w219 w226 w232 w235 w243 w251 w258 w267 w272 w295 w309] -> w94
      tunnel: w92 -> [_ _ _ _ _ _ _ _ _ _ _ _ _ _ _ _ _ _ _ w308]
      tunnel: w91 -> [_ w129 _ w163 _ _ w185 _ _ w218 _ w231 _ w244 _ w257 _ _ _ w306]
      tunnel: w90 -> [_ _ _ _ w167 _ _ _ _ _ _ _ _ _ _ _ _ _ _ w301]
      tunnel: w89 -> [_ _ _ _ w170 _ _ _ _ _ _ _ _ _ _ _ _ _ _ _]
      tunnel: w88 -> [_ _ _ _ w169 _ _ _ _ _ _ _ _ _ _ _ _ _ _ _]
      frame "Initalize", Default {
        w108 = T10 {"ENABLED"=FALSE, "High Limit (C)"=nan, "Low Limit (C)"=nan} ("Temperature 1 Alarm Setup")
        w110 = T25."Disabled and Grayed Out" ("Disabled")
        w114 = T25."Disabled and Grayed Out" ("Disabled")
        w115 = T25."Disabled and Grayed Out" ("Disabled")
        w116 = T25."Disabled and Grayed Out" ("Disabled")
        w117 = T25."Enabled" ("Disabled")
        w124 = dbl[][] [] ("Currents 2")
        n50 = local write "Running?"(FALSE ("Running?")) -> ()
        n51 = property on="START EXPERIMENT" class="Bool (strict)"("Value"=FALSE ("START EXPERIMENT")) -> ()  [unwired: 2 in, 2 out]
        n52 = property on="Tab Control" class="TabCtl (strict)"("Value"=enum32{"Overview", "Experiment", "Alarms"}."Overview" ("Tab Control")) -> ()  [unwired: 2 in, 2 out]
        n53 = Get Date/Time In Seconds() -> (seconds since 1Jan1904=w125:timestamp)
        n54 = To Double Precision Float(number=w125) -> (double precision float=w123:dbl)
        n55 = property on="Overview Temperatures" class="WFChart (strict)"("Value"=w124, "History Data"=w124, "XScale.Offset"=w123) -> ()  [unwired: 2 in, 2 out]
        n56 = property on="Overview Currents" class="WFChart (strict)"("Value"=w124, "History Data"=w124, "XScale.Offset"=w123) -> ()  [unwired: 2 in, 2 out]
        n57 = property on="Overview Voltages" class="WFChart (strict)"("Value"=0.0 ("Overview Voltages"), "History Data"=dbl[] [], "XScale.Offset"=w123) -> ()  [unwired: 2 in, 2 out]
        n58 = property on="START EXPERIMENT" class="Bool (strict)"("DisabledEnum"=w116) -> ()  [unwired: 2 in, 2 out]
        n59 = property on="DONE" class="Bool"("DisabledEnum"=T25."Enabled" ("Disabled")) -> ()  [unwired: 2 in, 2 out]
        n60 = property on="OPEN EXPERIMENT" class="Bool"("DisabledEnum"=w117) -> ()  [unwired: 2 in, 2 out]
        n61 = property on="NEW EXPERIMENT" class="Bool"("DisabledEnum"=w117) -> ()  [unwired: 2 in, 2 out]
        n62 = property on="CLOSE EXPERIMENT" class="Bool"("DisabledEnum"=w116) -> ()  [unwired: 2 in, 2 out]
        n63 = property on="SAVE EXPERIMENT" class="Bool"("DisabledEnum"=w116) -> ()  [unwired: 2 in, 2 out]
        n64 = local write "Temperature 1 Alarm Setup"(w108) -> ()
        n65 = local write "Temperature 2 Alarm Setup"(w108) -> ()
        n66 = local write "Temperature 3 Alarm Setup"(w108) -> ()
        n67 = local write "Average Temperature Alarm Setup"(w108) -> ()
        n68 = local write "Experiment Completed"(nan ("Experiment Completed")) -> ()
        n69 = local write "Experiment Total Runs"(u32 0 ("Experiment Total Runs")) -> ()
        n70 = local write "Runs"(T2[] [] ("Runs")) -> ()
        n71 = Enqueue Element(queue=w106, element=T23 {"Action"=enum."Read Alarm Controls", "Data"=variant}, error in (no error)=w105) -> (error out=w104:errorcluster)  [unwired: 1 in, 2 out]
        n72 = property on="Experiment Operator" class="Str"("DisabledEnum"=w114) -> ()  [unwired: 2 in, 2 out]
        n73 = property on="Experiment Project" class="Str"("DisabledEnum"=w114) -> ()  [unwired: 2 in, 2 out]
        n74 = property on="Experiment Target Dose (dpa)" class="DigNum (strict)"("DisabledEnum"=w114) -> ()  [unwired: 2 in, 2 out]
        n75 = property on="Experiment Sample Density (g/cm^3)" class="DigNum (strict)"("DisabledEnum"=w110) -> ()  [unwired: 2 in, 2 out]
        n76 = property on="Experiment Sample Description" class="Str"("DisabledEnum"=w110) -> ()  [unwired: 2 in, 2 out]
        n77 = property on="Experiment Sample Molar Mass (g/mol)" class="DigNum (strict)"("DisabledEnum"=w110) -> ()  [unwired: 2 in, 2 out]
        n78 = property on="Experiment Sample Irradiation Area (cm^2)" class="DigNum (strict)"("DisabledEnum"=w110) -> ()  [unwired: 2 in, 2 out]
        n79 = property on="Experiment Sample Name" class="Str"("DisabledEnum"=w110) -> ()  [unwired: 2 in, 2 out]
        n80 = property on="Experiment Sample SRIM Damage Peak (disp * ion / cm)" class="DigNum (strict)"("DisabledEnum"=w110) -> ()  [unwired: 2 in, 2 out]
        n81 = property on="SELECT SRIM" class="Bool"("DisabledEnum"=w110) -> ()  [unwired: 2 in, 2 out]
        n82 = property on="SHOW RUNS" class="Bool"("DisabledEnum"=w110) -> ()  [unwired: 2 in, 2 out]
        n83 = property on="Experiment Beam Line Charge State" class="DigNum (strict)"("DisabledEnum"=w115) -> ()  [unwired: 2 in, 2 out]
        n84 = property on="Experiment Beam Line Ion" class="Enum (strict)"("DisabledEnum"=w115) -> ()  [unwired: 2 in, 2 out]
        n85 = property on="Experiment Beam Line Type" class="Enum (strict)"("DisabledEnum"=w115) -> ()  [unwired: 2 in, 2 out]
        n86 = property on="Experiment Beam Line Total Source Ion Energy (kV)" class="DigNum (strict)"("DisabledEnum"=w115) -> ()  [unwired: 2 in, 2 out]
        n87 = Unbundle By Name(w104) -> ("status"=w107:bool)
      }
      frame "Create Experiment" {
        n88 = Bundle By Name(cluster=T26 {"Action"=enum."Create", "Data"=variant} ("element"), "Data"=w126) -> (w127:T26)
        n89 = Enqueue Element(queue=w129, element=w127) -> ()  [unwired: 2 in, 3 out]
      }
      frame "Created" {
        w132 = T25."Enabled" ("Disabled")
        w135 = T25."Enabled" ("Disabled")
        w136 = T25."Enabled" ("Disabled")
        w134 = T25."Enabled" ("Disabled")
        n90 = property on="Experiment Beam Line Charge State" class="DigNum (strict)"("DisabledEnum"=w135) -> ()  [unwired: 2 in, 2 out]
        n91 = property on="Experiment Beam Line Ion" class="Enum (strict)"("DisabledEnum"=w135) -> ()  [unwired: 2 in, 2 out]
        n92 = property on="Experiment Beam Line Type" class="Enum (strict)"("DisabledEnum"=w135) -> ()  [unwired: 2 in, 2 out]
        n93 = property on="Experiment Beam Line Total Source Ion Energy (kV)" class="DigNum (strict)"("DisabledEnum"=w135) -> ()  [unwired: 2 in, 2 out]
        n94 = property on="Experiment Operator" class="Str"("DisabledEnum"=w136) -> ()  [unwired: 2 in, 2 out]
        n95 = property on="Experiment Project" class="Str"("DisabledEnum"=w136) -> ()  [unwired: 2 in, 2 out]
        n96 = property on="Experiment Target Dose (dpa)" class="DigNum (strict)"("DisabledEnum"=w136) -> ()  [unwired: 2 in, 2 out]
        n97 = property on="CLOSE EXPERIMENT" class="Bool"("DisabledEnum"=w134) -> ()  [unwired: 2 in, 2 out]
        n98 = property on="START EXPERIMENT" class="Bool (strict)"("DisabledEnum"=w134) -> ()  [unwired: 2 in, 2 out]
        n99 = property on="SAVE EXPERIMENT" class="Bool"("DisabledEnum"=w134) -> ()  [unwired: 2 in, 2 out]
        n100 = property on="Experiment Sample Density (g/cm^3)" class="DigNum (strict)"("DisabledEnum"=w132) -> ()  [unwired: 2 in, 2 out]
        n101 = property on="Experiment Sample Description" class="Str"("DisabledEnum"=w132) -> ()  [unwired: 2 in, 2 out]
        n102 = property on="Experiment Sample Irradiation Area (cm^2)" class="DigNum (strict)"("DisabledEnum"=w132) -> ()  [unwired: 2 in, 2 out]
        n103 = property on="Experiment Sample Molar Mass (g/mol)" class="DigNum (strict)"("DisabledEnum"=w132) -> ()  [unwired: 2 in, 2 out]
        n104 = property on="Experiment Sample Name" class="Str"("DisabledEnum"=w132) -> ()  [unwired: 2 in, 2 out]
        n105 = property on="Experiment Sample SRIM Damage Peak (disp * ion / cm)" class="DigNum (strict)"("DisabledEnum"=w132) -> ()  [unwired: 2 in, 2 out]
        n106 = property on="SELECT SRIM" class="Bool"("DisabledEnum"=w132) -> ()  [unwired: 2 in, 2 out]
        n107 = property on="NEW EXPERIMENT" class="Bool"("DisabledEnum"=w134) -> ()  [unwired: 2 in, 2 out]
        n108 = property on="SHOW RUNS" class="Bool"("DisabledEnum"=w132) -> ()  [unwired: 2 in, 2 out]
      }
      frame "Read Experiment Controls" {
        n109 = local read "Experiment File Path"() -> (w141:path)
        n110 = Bundle By Name(cluster=T31 {"Name"="", "Description"="", "Molar Mass (g/mol)"=0.0, "Density (g/cm^3)"=0.0, "Irradiation Area (cm^2)"=0.0, "SRIM Damage Peak (disp * ions/cm)"=0.0} ("Sample"), "Name"="Experiment Sample Name", "Description"="Experiment Sample Description", "Molar Mass (g/mol)"="Experiment Sample Molar Mass (g/mol)", "Density (g/cm^3)"="Experiment Sample Density (g/cm^3)", "Irradiation Area (cm^2)"="Experiment Sample Irradiation Area (cm^2)", "SRIM Damage Peak (disp * ions/cm)"="Experiment Sample SRIM Damage Peak (disp * ion / cm)") -> (w150:T31)
        n111 = Bundle By Name(cluster=T28 {"Type"=enum."Ion Beam Analysis", "Ion"=enum."H", "Charge State"=0, "Total Source Ion Energy (kV)"=0.0} ("Beam Line"), "Type"="Experiment Beam Line Type", "Ion"="Experiment Beam Line Ion", "Charge State"="Experiment Beam Line Charge State", "Total Source Ion Energy (kV)"="Experiment Beam Line Total Source Ion Energy (kV)") -> (w145:T28)
        n112 = local read "Runs"() -> (w138:T2[])
        n113 = Bundle By Name(cluster=T32 {"File Path"=path "", "Operator"="", "Project"="", "Target Dose (dpa)"=0.0, "Sample"={"Name"="", "Description"="", "Molar Mass (g/mol)"=0.0, "Density (g/cm^3)"=0.0, "Irradiation Area (cm^2)"=0.0, "SRIM Damage Peak (disp * ions/cm)"=0.0}, "Beam Line"={"Type"=enum."Ion Beam Analysis", "Ion"=enum."H", "Charge State"=0, "Total Source Ion Energy (kV)"=0.0}, "Runs"=[]} ("Experiment"), "File Path"=w141, "Operator"="Experiment Operator", "Project"="Experiment Project", "Target Dose (dpa)"="Experiment Target Dose (dpa)", "Sample"=w150, "Beam Line"=w145, "Runs"=w138) -> (w159:T32)
        n114 = To Variant(anything=w159) -> (Variant=w161:variant)
        n115 = Bundle By Name(cluster=T26 {"Action"=enum."Load", "Data"=variant} ("element"), "Data"=w161) -> (w143:T26)
        n116 = Enqueue Element(queue=w163, element=w143) -> ()  [unwired: 2 in, 3 out]
      }
      frame "Read Alarm Controls" {
        # "Need to flush the queue to remove any \"Check\" commands that will check for an alarm based on the old setups and not the new setups. This also disables the alarms much faster."
        n117 = Build Array("Temperature 1 Alarm Setup", "Temperature 2 Alarm Setup", "Temperature 3 Alarm Setup", "Average Temperature Alarm Setup") -> (w165:T10[])
        n118 = Bundle By Name(cluster=T35 {"Temperature"=[]} ("Alarm Setups"), "Temperature"=w165) -> (w174:T35)
        n119 = call "SetAlarmControlState.vi"("Low Limit Control Ref"=w169, "High Limit Control Ref"=w170, "Alarm Setups"=w165) -> ()  [unwired: 8 in, 1 out]
        n120 = To Variant(anything=w174) -> (Variant=w172:variant)
        n121 = Bundle By Name(cluster=T33 {"Action"=enum."Load", "Data"=variant} ("Alarm Queue Element"), "Data"=w172) -> (w171:T33)
        n122 = Flush Queue(queue=w167) -> (queue out=w168:refnum<queue>, error out=w166:errorcluster)  [unwired: 1 in, 1 out]
        n123 = Enqueue Element(queue=w168, element=w171, error in (no error)=w166) -> ()  [unwired: 1 in, 3 out]
      }
      frame "Loaded" {
      }
      frame "Save Experiment" {
        n124 = Enqueue Element(queue=w185, element=T26 {"Action"=enum."Save", "Data"=variant}) -> ()  [unwired: 2 in, 3 out]
      }
      frame "Saved" {
      }
      frame "Write Experiment Controls" {
        n125 = Variant To Data(type=T32 {"File Path"=path "", "Operator"="Operator", "Project"="Project Description", "Target Dose (dpa)"=0.0, "Sample"={"Name"="", "Description"="", "Molar Mass (g/mol)"=0.0, "Density (g/cm^3)"=0.0, "Irradiation Area (cm^2)"=0.0, "SRIM Damage Peak (disp * ions/cm)"=0.0}, "Beam Line"={"Type"=enum."Ion Beam Analysis", "Ion"=enum."H", "Charge State"=0, "Total Source Ion Energy (kV)"=nan}, "Runs"=[]} ("Experiment"), Variant=w198) -> (data=w193:T32)  [unwired: 1 in, 1 out]
        n126 = Unbundle By Name(w193) -> ("File Path"=→"Experiment File Path":path, "Operator"=w211:string, "Project"=w208:string, "Target Dose (dpa)"=w210:dbl, "Sample"=w209:T31, "Beam Line"=w201:T28, "Runs"=→"Runs":T2[])
        n127 = call "GetExperimentCompleted.vi"("Experiment"=w193) -> ("Total Runs"=→"Experiment Total Runs":i32, "Experiment Completed (%)"=w190:dbl)  [unwired: 9 in]
        n128 = Unbundle By Name(w209) -> ("Name"=w207:string, "Description"=w206:string, "Molar Mass (g/mol)"=w205:dbl, "Density (g/cm^3)"=w204:dbl, "Irradiation Area (cm^2)"=w203:dbl, "SRIM Damage Peak (disp * ions/cm)"=w202:dbl)
        n129 = Unbundle By Name(w201) -> ("Type"=w195:T29, "Ion"=w194:T30, "Charge State"=w200:u8, "Total Source Ion Energy (kV)"=w199:dbl)
        n130 = local write "Experiment Completed"(w190) -> ()
        n131 = local write "Experiment Operator"(w211) -> ()
        n132 = local write "Experiment Project"(w208) -> ()
        n133 = local write "Experiment Target Dose (dpa)"(w210) -> ()
        n134 = local write "Experiment Sample Name"(w207) -> ()
        n135 = local write "Experiment Sample Description"(w206) -> ()
        n136 = local write "Experiment Sample Molar Mass (g/mol)"(w205) -> ()
        n137 = local write "Experiment Sample Density (g/cm^3)"(w204) -> ()
        n138 = local write "Experiment Sample Irradiation Area (cm^2)"(w203) -> ()
        n139 = local write "Experiment Sample SRIM Damage Peak (disp * ion / cm)"(w202) -> ()
        n140 = local write "Experiment Beam Line Type"(w195) -> ()
        n141 = local write "Experiment Beam Line Ion"(w194) -> ()
        n142 = local write "Experiment Beam Line Charge State"(w200) -> ()
        n143 = local write "Experiment Beam Line Total Source Ion Energy (kV)"(w199) -> ()
      }
      frame "Read Experiment" {
        n144 = Variant To Data(type=path "", Variant=w221) -> (data=w215:path)  [unwired: 1 in, 1 out]
        n145 = To Variant(anything=w215) -> (Variant=w216:variant)
        n146 = Bundle By Name(cluster=T26 {"Action"=enum."Read", "Data"=variant} ("element"), "Data"=w216) -> (w214:T26)
        n147 = Enqueue Element(queue=w218, element=w214) -> ()  [unwired: 2 in, 3 out]
      }
      frame "Read" {
        n148 = Bundle By Name(cluster=T23 {"Action"=enum."Created", "Data"=variant} ("element"), "Data"=w224) -> (w223:T23)
        n149 = Enqueue Element(queue=w228, element=w223, error in (no error)=w227) -> (error out=w226:errorcluster)  [unwired: 1 in, 2 out]
      }
      frame "Start Experiment" {
        n150 = Enqueue Element(queue=w231, element=T26 {"Action"=enum."Start", "Data"=variant}) -> ()  [unwired: 2 in, 3 out]
      }
      frame "Started" {
        w236 = T25."Disabled and Grayed Out" ("Disabled")
        w237 = T25."Disabled and Grayed Out" ("Disabled")
        w238 = T25."Disabled and Grayed Out" ("Disabled")
        w239 = T25."Disabled and Grayed Out" ("Disabled")
        n151 = property on="DONE" class="Bool"("DisabledEnum"=T25."Disabled and Grayed Out" ("Disabled")) -> ()  [unwired: 2 in, 2 out]
        n152 = property on="Experiment Sample Density (g/cm^3)" class="DigNum (strict)"("DisabledEnum"=w237) -> ()  [unwired: 2 in, 2 out]
        n153 = property on="Experiment Sample Description" class="Str"("DisabledEnum"=w237) -> ()  [unwired: 2 in, 2 out]
        n154 = property on="Experiment Sample Irradiation Area (cm^2)" class="DigNum (strict)"("DisabledEnum"=w237) -> ()  [unwired: 2 in, 2 out]
        n155 = property on="Experiment Sample Molar Mass (g/mol)" class="DigNum (strict)"("DisabledEnum"=w237) -> ()  [unwired: 2 in, 2 out]
        n156 = property on="Experiment Sample Name" class="Str"("DisabledEnum"=w237) -> ()  [unwired: 2 in, 2 out]
        n157 = property on="Experiment Sample SRIM Damage Peak (disp * ion / cm)" class="DigNum (strict)"("DisabledEnum"=w237) -> ()  [unwired: 2 in, 2 out]
        n158 = property on="SELECT SRIM" class="Bool"("DisabledEnum"=w237) -> ()  [unwired: 2 in, 2 out]
        n159 = property on="SAVE EXPERIMENT" class="Bool"("DisabledEnum"=w239) -> ()  [unwired: 2 in, 2 out]
        n160 = property on="OPEN EXPERIMENT" class="Bool"("DisabledEnum"=w239) -> ()  [unwired: 2 in, 2 out]
        n161 = property on="CLOSE EXPERIMENT" class="Bool"("DisabledEnum"=w239) -> ()  [unwired: 2 in, 2 out]
        n162 = property on="NEW EXPERIMENT" class="Bool"("DisabledEnum"=w239) -> ()  [unwired: 2 in, 2 out]
        n163 = property on="Experiment Operator" class="Str"("DisabledEnum"=w236) -> ()  [unwired: 2 in, 2 out]
        n164 = property on="Experiment Project" class="Str"("DisabledEnum"=w236) -> ()  [unwired: 2 in, 2 out]
        n165 = property on="Experiment Target Dose (dpa)" class="DigNum (strict)"("DisabledEnum"=w236) -> ()  [unwired: 2 in, 2 out]
        n166 = property on="Experiment Beam Line Charge State" class="DigNum (strict)"("DisabledEnum"=w238) -> ()  [unwired: 2 in, 2 out]
        n167 = property on="Experiment Beam Line Type" class="Enum (strict)"("DisabledEnum"=w238) -> ()  [unwired: 2 in, 2 out]
        n168 = property on="Experiment Beam Line Ion" class="Enum (strict)"("DisabledEnum"=w238) -> ()  [unwired: 2 in, 2 out]
        n169 = property on="Experiment Beam Line Total Source Ion Energy (kV)" class="DigNum (strict)"("DisabledEnum"=w238) -> ()  [unwired: 2 in, 2 out]
        "Running?" <- TRUE ("Running?")
      }
      frame "Stop Experiment" {
        n170 = Enqueue Element(queue=w244, element=T26 {"Action"=enum."Stop", "Data"=variant}) -> ()  [unwired: 2 in, 3 out]
      }
      frame "Stopped" {
        w253 = FALSE ("START EXPERIMENT")
        w246 = T25."Enabled" ("Disabled")
        n171 = local write "Running?"(w253) -> ()
        n172 = local write "START EXPERIMENT"(w253) -> ()
        n173 = Bundle By Name(cluster=T23 {"Action"=enum."Created", "Data"=variant} ("element"), "Data"=w248) -> (w247:T23)
        n174 = Enqueue Element(queue=w252, element=w247, error in (no error)=w250) -> (error out=w251:errorcluster)  [unwired: 1 in, 2 out]
        n175 = property on="OPEN EXPERIMENT" class="Bool"("DisabledEnum"=w246) -> ()  [unwired: 2 in, 2 out]
        n176 = property on="NEW EXPERIMENT" class="Bool"("DisabledEnum"=w246) -> ()  [unwired: 2 in, 2 out]
        n177 = property on="DONE" class="Bool"("DisabledEnum"=T25."Enabled" ("Disabled")) -> ()  [unwired: 2 in, 2 out]
      }
      frame "Close Experiment" {
        n178 = Enqueue Element(queue=w257, element=T26 {"Action"=enum."Initialize", "Data"=variant}) -> ()  [unwired: 2 in, 3 out]
      }
      frame "Closed" {
        w260 = T25."Disabled and Grayed Out" ("Disabled")
        w261 = T25."Disabled and Grayed Out" ("Disabled")
        w262 = T25."Disabled and Grayed Out" ("Disabled")
        w263 = T25."Disabled and Grayed Out" ("Disabled")
        n179 = property on="Experiment Operator" class="Str"("DisabledEnum"=w262) -> ()  [unwired: 2 in, 2 out]
        n180 = property on="Experiment Project" class="Str"("DisabledEnum"=w262) -> ()  [unwired: 2 in, 2 out]
        n181 = property on="Experiment Target Dose (dpa)" class="DigNum (strict)"("DisabledEnum"=w262) -> ()  [unwired: 2 in, 2 out]
        n182 = Bundle By Name(cluster=T23 {"Action"=enum."Write Experiment Controls", "Data"=variant} ("element"), "Data"=w265) -> (w264:T23)
        n183 = Enqueue Element(queue=w269, element=w264, error in (no error)=w268) -> (error out=w267:errorcluster)  [unwired: 1 in, 2 out]
        n184 = property on="CLOSE EXPERIMENT" class="Bool"("DisabledEnum"=w263) -> ()  [unwired: 2 in, 2 out]
        n185 = property on="SAVE EXPERIMENT" class="Bool"("DisabledEnum"=w263) -> ()  [unwired: 2 in, 2 out]
        n186 = property on="START EXPERIMENT" class="Bool (strict)"("DisabledEnum"=w263) -> ()  [unwired: 2 in, 2 out]
        n187 = property on="Experiment Beam Line Charge State" class="DigNum (strict)"("DisabledEnum"=w261) -> ()  [unwired: 2 in, 2 out]
        n188 = property on="Experiment Beam Line Ion" class="Enum (strict)"("DisabledEnum"=w261) -> ()  [unwired: 2 in, 2 out]
        n189 = property on="Experiment Beam Line Type" class="Enum (strict)"("DisabledEnum"=w261) -> ()  [unwired: 2 in, 2 out]
        n190 = property on="Experiment Beam Line Total Source Ion Energy (kV)" class="DigNum (strict)"("DisabledEnum"=w261) -> ()  [unwired: 2 in, 2 out]
        n191 = property on="Experiment Sample Density (g/cm^3)" class="DigNum (strict)"("DisabledEnum"=w260) -> ()  [unwired: 2 in, 2 out]
        n192 = property on="Experiment Sample Description" class="Str"("DisabledEnum"=w260) -> ()  [unwired: 2 in, 2 out]
        n193 = property on="Experiment Sample Irradiation Area (cm^2)" class="DigNum (strict)"("DisabledEnum"=w260) -> ()  [unwired: 2 in, 2 out]
        n194 = property on="Experiment Sample Molar Mass (g/mol)" class="DigNum (strict)"("DisabledEnum"=w260) -> ()  [unwired: 2 in, 2 out]
        n195 = property on="Experiment Sample Name" class="Str"("DisabledEnum"=w260) -> ()  [unwired: 2 in, 2 out]
        n196 = property on="Experiment Sample SRIM Damage Peak (disp * ion / cm)" class="DigNum (strict)"("DisabledEnum"=w260) -> ()  [unwired: 2 in, 2 out]
        n197 = property on="SELECT SRIM" class="Bool"("DisabledEnum"=w260) -> ()  [unwired: 2 in, 2 out]
        n198 = property on="SHOW RUNS" class="Bool"("DisabledEnum"=w260) -> ()  [unwired: 2 in, 2 out]
      }
      frame "SRIM" {
        n199 = Variant To Data(type=path "", Variant=w279) -> (data=w277:path, error out=w276:errorcluster)  [unwired: 1 in]
        n200 = call "SRIMDialog.vi"("Error In"=w276, "SRIM Simulation File Path"=w277) -> ("Error Out"=w275:errorcluster, "SRIM Damage Peak D1 (disp * ion / cm)"=w274:dbl)  [unwired: 7 in, 1 out]
        n201 = case shown="No Error" w275 {
          selector: w275 -> [_ w285]
          tunnel: w274 -> [w282 _]
          tunnel: w273 -> [w281 w288]
          tunnel: [w281 w287] -> w272
          tunnel: w271 -> [_ w289]
          frame No Error {
            n202 = local write "Experiment Sample SRIM Damage Peak (disp * ion / cm)"(w282) -> ()
          }
          frame Error {
            n203 = To Variant(anything=w285) -> (Variant=w284:variant)
            n204 = Bundle By Name(cluster=T23 {"Action"=enum."Error", "Data"=variant} ("element"), "Data"=w284) -> (w283:T23)
            n205 = Enqueue Element(queue=w289, element=w283, error in (no error)=w288) -> (error out=w287:errorcluster)  [unwired: 1 in, 2 out]
          }
        }
      }
      frame "Error" {
        w293 = T39 1 items=["no dialog", "OK message", "continue or stop message", "OK message + warnings", "continue/stop + warnings"] ("type of dialog (OK msg:1)")
        n206 = Variant To Data(type=w295, Variant=w296) -> (data=w294:errorcluster)  [unwired: 1 in, 1 out]
        n207 = call <vilib>:"General Error Handler.vi"("[user-defined codes]"=i32[] [5000, 5001, 5002, 5003, 5004, 5005, 5006], "[user-defined descriptions]"=string[] ["An operator name must be entered. The operator cannot be blank or \"Operator\".", "The \"Target Dose\" cannot be zero or Not a Number (NaN).", "The \"Molar Mass\" for the sample cannot be zero or Not a Number (NaN).", "The \"Density\" for the sample cannot be zero or Not a Number (NaN).", "The \"Irradiation Area\" for the sample cannot be zero or Not a Number (NaN).", "The \"SRIM Damage PeaK\" for the sample cannot be zero or Not a Number (NaN).", "The \"Total Source Ion Energy\" for the beam line cannot be zero or Not a Number (NaN)."], "type of dialog (OK msg:1)"=w293, "error in (no error)"=w294) -> ()  [unwired: 7 in, 5 out]
        n208 = local write "START EXPERIMENT"(FALSE ("START EXPERIMENT")) -> ()
      }
      frame "Shutdown" {
        w315 = dbl[][] [] ("Currents 2")
        # "Flush the action queues so shutdown occurs almost immediately. Otherwise, all of the queue will have empty before shutdown occurs."
        n209 = Flush Queue(queue=w301) -> (queue out=w300:refnum<queue>, error out=w299:errorcluster)  [unwired: 1 in, 1 out]
        n210 = Flush Queue(queue=w306) -> (queue out=w305:refnum<queue>, error out=w304:errorcluster)  [unwired: 1 in, 1 out]
        n211 = Flush Queue(queue=w308) -> (queue out=w307:refnum<queue>, error out=w303:errorcluster)  [unwired: 1 in, 1 out]
        n212 = Not(x=w320) -> (.not. x?=w319:bool)
        n213 = Release Queue(queue=w311, error in (no error)=w310) -> (error out=w309:errorcluster)  [unwired: 1 in, 2 out]
        n214 = Enqueue Element(queue=w300, element=T33 {"Action"=enum."Shutdown", "Data"=variant}, error in (no error)=w299) -> ()  [unwired: 1 in, 3 out]
        n215 = Enqueue Element(queue=w307, element=T37 {"Action"=enum."Shutdown", "Data"=variant} ("Hardware Queue Element"), error in (no error)=w303) -> ()  [unwired: 1 in, 3 out]
        n216 = Enqueue Element(queue=w305, element=T26 {"Action"=enum."Shutdown", "Data"=variant}, error in (no error)=w304) -> ()  [unwired: 1 in, 3 out]
        n217 = property on="DONE" class="Bool"("DisabledEnum"=T25."Enabled" ("Disabled")) -> ()  [unwired: 2 in, 2 out]
        n218 = Get Date/Time In Seconds() -> (seconds since 1Jan1904=w316:timestamp)
        n219 = To Double Precision Float(number=w316) -> (double precision float=w314:dbl)
        n220 = property on="Overview Currents" class="WFChart (strict)"("Value"=w315, "History Data"=w315, "XScale.Offset"=w314) -> ()  [unwired: 2 in, 2 out]
        n221 = property on="Overview Temperatures" class="WFChart (strict)"("Value"=w315, "History Data"=w315, "XScale.Offset"=w314) -> ()  [unwired: 2 in, 2 out]
        n222 = property on="Overview Voltages" class="WFChart (strict)"("Value"=0.0 ("Overview Voltages"), "History Data"=dbl[] [], "XScale.Offset"=w314) -> ()  [unwired: 2 in, 2 out]
      }
    }
  }
  n223 = while "BPM Display Loop" {
    tunnel: w23 -> [w321]
    stop <- w322 stop-if-true
    # "The beam profile is relatively quick and no need to update other hardware indicators so fast. Thus, the BPM has its own display loop."
    n224 = Wait on Notification(notifier=w321) -> (notification=→"Beam Profile":T40, error out=w322:errorcluster)  [unwired: 3 in, 2 out]
  }
  n225 = while "UI Event Loop" {
    tunnel: w33 -> [w329]
    shift-right: [w327] -> w31
    shift-left: w17 -> [w324]
    tunnel: w27 -> [w326]
    tunnel: w4 -> [w325]
    stop <- w328 stop-if-true
    # "The UI Event Loop simply passes actions to the UI Action loop based on UI events"
    n226 = case shown="No Error" w324 {
      selector: w324 -> [w330 w495]
      tunnel: w329 -> [w335 w494]
      tunnel: [w334 w493] -> w328
      tunnel: [w333 w495] -> w327
      tunnel: w326 -> [w332 _]
      tunnel: w325 -> [w331 _]
      frame No Error {
        n227 = event shown="[4] \"NEW EXPERIMENT\": Value Change" {
          selector: _ -> [_ _ _ _ _ _ _ _ _ _ _ _ _ _ _]
          dyn-events: _ -> [_ _ _ _ _ _ _ _ _ _ _ _ _ _ _]
          timeout: _ -> [_ _ _ _ _ _ _ _ _ _ _ _ _ _ _]
          tunnel: w335 -> [w337 w346 w362 w371 w393 w417 w427 w431 w434 w437 w441 w466 w478 w489 w491]
          tunnel: [w337 w345 w361 w371 w393 w417 w427 w431 w434 w437 w441 w466 w478 w489 w491] -> w334
          tunnel: w330 -> [w336 w341 w355 w374 w392 w410 w428 w433 w435 w438 w445 w464 w476 w488 w492]
          tunnel: [w336 w344 w360 w372 w388 w409 w428 w432 w435 w438 w442 w463 w475 w488 w492] -> w333
          tunnel: w332 -> [_ w342 w358 w373 w389 w408 _ w430 _ _ w446 w465 w477 _ _]
          tunnel: w331 -> [_ _ _ _ w394 w416 _ _ _ _ w447 _ w474 _ _]
          event Timeout {
            n228 = event-data() -> ()  [unwired: 1 in, 2 out]
          }
          event Panel Close? {
            n229 = event-data() -> ()  [unwired: 1 in, 3 out]
            n230 = Not(x=w346) -> (.not. x?=w345:bool)
            n231 = local read "Running?"() -> (w338:bool)
            n232 = case shown="True" w338 {
              tunnel: w342 -> [w348 w353]
              tunnel: [w348 w352] -> w339
              tunnel: [w347 w351] -> w340
              tunnel: w341 -> [w347 w350]
              frame False {
              }
              frame True {
                n233 = Enqueue Element(queue=w353, element=T23 {"Action"=enum."Stop Experiment", "Data"=variant}, error in (no error)=w350) -> (queue out=w352:refnum<queue>, error out=w351:errorcluster)  [unwired: 1 in, 1 out]
              }
            }
            n234 = Enqueue Element(queue=w339, element=T23 {"Action"=enum."Shutdown", "Data"=variant} ("User Interface Queue Element"), error in (no error)=w340) -> (error out=w344:errorcluster)  [unwired: 1 in, 2 out]
            n235 = event-data("Discard?"=w345) -> ()  [unwired: 1 in, 1 out]
          }
          event "DONE": Value Change {
            n236 = event-data() -> ()  [unwired: 1 in, 5 out]
            n237 = Not(x=w362) -> (.not. x?=w361:bool)
            n238 = local read "Running?"() -> (w354:bool)
            n239 = case shown="True" w354 {
              tunnel: w358 -> [w364 w369]
              tunnel: [w364 w368] -> w357
              tunnel: [w363 w367] -> w356
              tunnel: w355 -> [w363 w366]
              frame False {
              }
              frame True {
                n240 = Enqueue Element(queue=w369, element=T23 {"Action"=enum."Stop Experiment", "Data"=variant}, error in (no error)=w366) -> (queue out=w368:refnum<queue>, error out=w367:errorcluster)  [unwired: 1 in, 1 out]
              }
            }
            n241 = Enqueue Element(queue=w357, element=T23 {"Action"=enum."Shutdown", "Data"=variant}, error in (no error)=w356) -> (error out=w360:errorcluster)  [unwired: 1 in, 2 out]
          }
          event "START EXPERIMENT": Value Change {
            n242 = event-data() -> ()  [unwired: 1 in, 1 out]
            n243 = case shown="True" "START EXPERIMENT" {
              tunnel: w374 -> [w377 w385]
              tunnel: w373 -> [w378 w384]
              tunnel: [w376 w380] -> w372
              frame False {
                n244 = Enqueue Element(queue=w378, element=T23 {"Action"=enum."Stop Experiment", "Data"=variant}, error in (no error)=w377) -> (error out=w376:errorcluster)  [unwired: 1 in, 2 out]
              }
              frame True {
                n245 = Enqueue Element(queue=w384, element=T23 {"Action"=enum."Read Experiment Controls", "Data"=variant}, error in (no error)=w385) -> (queue out=w382:refnum<queue>, error out=w381:errorcluster)  [unwired: 1 in, 1 out]
                n246 = Enqueue Element(queue=w382, element=T23 {"Action"=enum."Start Experiment", "Data"=variant}, error in (no error)=w381) -> (error out=w380:errorcluster)  [unwired: 1 in, 2 out]
              }
            }
          }
          event "NEW EXPERIMENT": Value Change {
            n247 = event-data() -> ()  [unwired: 1 in, 5 out]
            n248 = Unbundle By Name(w394) -> ("Folder.Experiment"=w397:path)
            n249 = call "SelectFile.vi"("Button Label"="Create", "Prompt"="Create New Experiment File", "File Description"="Experiment File", "File Extension (.*)"=".xml", "Start Path"=w397) -> ("Cancelled?"=w391:bool, "Selected File Path"=w390:path)  [unwired: 4 in, 1 out]
            n250 = case shown="False" w391 {
              tunnel: w392 -> [w402 w405]
              tunnel: w390 -> [w404 _]
              tunnel: w389 -> [w403 _]
              tunnel: [w401 w405] -> w388
              frame False {
                n251 = To Variant(anything=w404) -> (Variant=w399:variant)
                n252 = Bundle By Name(cluster=T23 {"Action"=enum."Create Experiment", "Data"=variant} ("element"), "Data"=w399) -> (w398:T23)
                n253 = Enqueue Element(queue=w403, element=w398, error in (no error)=w402) -> (error out=w401:errorcluster)  [unwired: 1 in, 2 out]
              }
              frame True {
              }
            }
          }
          event "OPEN EXPERIMENT": Value Change {
            n254 = event-data() -> ()  [unwired: 1 in, 5 out]
            n255 = Unbundle By Name(w416) -> ("Folder.Experiment"=w415:path)
            n256 = call "SelectFile.vi"("Button Label"="Open", "Prompt"="Open Experiment File", "File Description"="Experiment File", "File Extension (.*)"=".xml", "Start Path"=w415) -> ("Cancelled?"=w412:bool, "Selected File Path"=w411:path)  [unwired: 4 in, 1 out]
            n257 = case shown="False" w412 {
              tunnel: w411 -> [w421 _]
              tunnel: w410 -> [w424 w425]
              tunnel: [w418 w425] -> w409
              tunnel: w408 -> [w423 _]
              frame False {
                n258 = To Variant(anything=w421) -> (Variant=w420:variant)
                n259 = Bundle By Name(cluster=T23 {"Action"=enum."Read Experiment", "Data"=variant} ("element"), "Data"=w420) -> (w419:T23)
                n260 = Enqueue Element(queue=w423, element=w419, error in (no error)=w424) -> (error out=w418:errorcluster)  [unwired: 1 in, 2 out]
              }
              frame True {
              }
            }
          }
          event "OVERVIEW": Value Change {
            n261 = event-data() -> ()  [unwired: 1 in, 1 out]
            n262 = property on="Tab Control" class="TabCtl (strict)"("Value"=enum32{"Overview", "Experiment", "Alarms"}."Overview" ("Tab Control")) -> ()  [unwired: 2 in, 2 out]
          }
          event Value Change {
            n263 = event-data() -> ()  [unwired: 1 in, 5 out]
            n264 = Enqueue Element(queue=w430, element=T23 {"Action"=enum."Read Alarm Controls", "Data"=variant}, error in (no error)=w433) -> (error out=w432:errorcluster)  [unwired: 1 in, 2 out]
          }
          event Value Change {
            n265 = event-data() -> ()  [unwired: 1 in, 5 out]
            n266 = call "AboutDialog.vi"() -> ()  [unwired: 11 in, 1 out]
          }
          event "EXPERIMENT": Value Change {
            n267 = event-data() -> ()  [unwired: 1 in, 5 out]
            n268 = property on="Tab Control" class="TabCtl (strict)"("Value"=enum32{"Overview", "Experiment", "Alarms"}."Experiment" ("Tab Control")) -> ()  [unwired: 2 in, 2 out]
          }
          event "SAVE EXPERIMENT": Value Change {
            n269 = event-data() -> ()  [unwired: 1 in, 5 out]
            n270 = Unbundle By Name(w447) -> ("Folder.Experiment Log"=w450:path)
            n271 = call "SelectFile.vi"("Button Label"="Save", "Prompt"="Save Experiment File", "File Description"="Experiment File", "File Extension (.*)"=".xml", "Start Path"=w450) -> ("Cancelled?"=w444:bool, "Selected File Path"=w443:path)  [unwired: 4 in, 1 out]
            n272 = case shown="False" w444 {
              tunnel: w446 -> [w458 _]
              tunnel: w445 -> [w457 w461]
              tunnel: w443 -> [w454 _]
              tunnel: [w451 w461] -> w442
              frame False {
                n273 = stacked-sequence {
                  tunnel: w454 -> [w460]
                  tunnel: [T23 {"Action"=enum."Read Experiment Controls", "Data"=variant} ("element")] -> w452
                  frame #0 {
                    n274 = local write "Experiment File Path"(w460) -> ()
                  }
                }
                n275 = Enqueue Element(queue=w458, element=w452, error in (no error)=w457) -> (queue out=w455:refnum<queue>, error out=w456:errorcluster)  [unwired: 1 in, 1 out]
                n276 = Enqueue Element(queue=w455, element=T23 {"Action"=enum."Save Experiment", "Data"=variant}, error in (no error)=w456) -> (error out=w451:errorcluster)  [unwired: 1 in, 2 out]
              }
              frame True {
              }
            }
          }
          event "CLOSE EXPERIMENT": Value Change {
            n277 = event-data() -> ()  [unwired: 1 in, 5 out]
            n278 = Enqueue Element(queue=w465, element=T23 {"Action"=enum."Close Experiment", "Data"=variant}, error in (no error)=w464) -> (error out=w463:errorcluster)  [unwired: 1 in, 2 out]
          }
          event "SELECT SRIM": Value Change {
            n279 = event-data() -> ()  [unwired: 1 in, 5 out]
            n280 = Unbundle By Name(w474) -> ("Folder.SRIM Simulation"=w473:path)
            n281 = call "SelectFile.vi"("Button Label"="Select", "Prompt"="Select SRIM Simulation File", "File Description"="SRIM Simulation File", "File Extension (.*)"=".txt", "Start Path"=w473) -> ("Cancelled?"=w470:bool, "Selected File Path"=w469:path)  [unwired: 4 in, 1 out]
            n282 = case shown="False" w470 {
              tunnel: w477 -> [w485 _]
              tunnel: w476 -> [w484 w486]
              tunnel: [w483 w486] -> w475
              tunnel: w469 -> [w480 _]
              frame False {
                n283 = To Variant(anything=w480) -> (Variant=w481:variant)
                n284 = Bundle By Name(cluster=T23 {"Action"=enum."SRIM", "Data"=variant} ("element"), "Data"=w481) -> (w479:T23)
                n285 = Enqueue Element(queue=w485, element=w479, error in (no error)=w484) -> (error out=w483:errorcluster)  [unwired: 1 in, 2 out]
              }
              frame True {
              }
            }
          }
          event "SHOW RUNS": Value Change {
            n286 = event-data() -> ()  [unwired: 1 in, 1 out]
            n287 = local read "Runs"() -> (w487:T2[])
            n288 = call "RunsDialog.vi"("Runs In"=w487) -> ()  [unwired: 10 in, 1 out]
          }
          event "ALARMS": Value Change {
            n289 = event-data() -> ()  [unwired: 1 in, 5 out]
            n290 = property on="Tab Control" class="TabCtl (strict)"("Value"=enum32{"Overview", "Experiment", "Alarms"}."Alarms" ("Tab Control")) -> ()  [unwired: 2 in, 2 out]
          }
        }
      }
      frame Error {
        n291 = Not(x=w494) -> (.not. x?=w493:bool)
      }
    }
  }
  n292 = call "HardwareLoop.vi"("Error In"=w17, "ABLE Configuration"=w4, "ABLE Data Structures"=w18, "Action Queues"=w19) -> ("Error Out"=w28:errorcluster)  [unwired: 7 in]
  n293 = call "AlarmLoop.vi"("Error In"=w17, "ABLE Configuration"=w4, "ABLE Data Structures"=w18, "Action Queues"=w19) -> ("Error Out"=w15:errorcluster)  [unwired: 7 in]
  n294 = call "ExperimentLoop.vi"("Error In"=w17, "ABLE Configuration"=w4, "ABLE Data Structures"=w18, "Action Queues"=w19) -> ("Error Out"=w16:errorcluster)  [unwired: 7 in]
  n295 = Merge Errors(w31, w30, w28, w15, w16) -> (w29:errorcluster)
  n296 = call "Shutdown.vi"("Error In"=w29) -> ()  [unwired: 11 in]
